vi "Motors help!.vi"(0 "Enable Motors":refnum<vi>, 1 "Cluster":T1, 2 "Motors Visa Ref":refnum<visa-resource-name>="COM7") -> ()   [LabVIEW 2010]
panel:
  out "theta-":refnum<vi>
  out "theta+":refnum<vi>
  out "Delta Theta (deg)":refnum<vi>
  out "Theta Speed (deg/s)":refnum<vi>
  out "theta-?":refnum<vi>
  out "theta+?":refnum<vi>
  out "Defined Positions":refnum<vi>
  out "Go To Saved Position?":refnum<vi>
  out "Saved Positions":refnum<vi>
  out "z-":refnum<vi>
  out "z+":refnum<vi>
  out "Delta Z (mm)":refnum<vi>
  out "Z Speed (mm/s)":refnum<vi>
  out "z-?":refnum<vi>
  out "z+?":refnum<vi>
  out "Y Speed (mm/s)":refnum<vi>
  out "y-":refnum<vi>
  out "y+":refnum<vi>
  out "Delta Y (mm)":refnum<vi>
  out "y-?":refnum<vi>
  out "y+?":refnum<vi>
  out "x-":refnum<vi>
  out "x+":refnum<vi>
  out "X Speed (mm/s)":refnum<vi>
  out "Delta X (mm)":refnum<vi>
  out "x-?":refnum<vi>
  out "x+?":refnum<vi>
  out "Jog-Mode":refnum<vi>
  out "Theta Go To":refnum<vi>
  out "Theta Go?":refnum<vi>
  out "Z Go To":refnum<vi>
  out "Z Go?":refnum<vi>
  out "Y Go To":refnum<vi>
  out "Y Go?":refnum<vi>
  out "X Go To":refnum<vi>
  out "X Go?":refnum<vi>
  out "Use Datums Nearest Hard Limits to Reset Origin?":refnum<vi>
  out "Saved Limits":refnum<vi>
  out "Find Datums Nearest Hard Limits?":refnum<vi>
  out "Theta Moving":refnum<vi>
  out "Status Theta":refnum<vi>
  out "Theta (deg)":refnum<vi>
  out "Theta Jogger Fast Speed":refnum<vi>
  out "Theta Jogger Normal Speed":refnum<vi>
  out "Theta Slew Speed (mm or degree/s)":refnum<vi>
  out "Z Moving":refnum<vi>
  out "Status Z":refnum<vi>
  out "Z-Axis (mm)":refnum<vi>
  out "Z Jogger Fast Speed":refnum<vi>
  out "Z Jogger Normal Speed":refnum<vi>
  out "Z Slew Speed (mm or degree/s)":refnum<vi>
  out "Y Moving":refnum<vi>
  out "Status Y":refnum<vi>
  out "Y-Axis (mm)":refnum<vi>
  out "Y Jogger Fast Speed":refnum<vi>
  out "Y Jogger Normal Speed":refnum<vi>
  out "Y Slew Speed (mm or degree/s)":refnum<vi>
  out "X Moving":refnum<vi>
  out "Status X":refnum<vi>
  out "X-Axis (mm)":refnum<vi>
  out "X Slew Speed (mm or degree/s)":refnum<vi>
  out "X Jogger Fast Speed":refnum<vi>
  out "X Jogger Normal Speed":refnum<vi>
  out "Set Jogger?":refnum<vi>
  out "Normal":refnum<vi>
  out "Fast":refnum<vi>
  out "Jogger Axis":refnum<vi>
  out "Theta Multiplier":refnum<vi>
  out "Z Multiplier":refnum<vi>
  out "Y Multiplier":refnum<vi>
  out "X Multiplier":refnum<vi>
  out "Need to Update Motor Parameters":refnum<vi>
  out "(degrees/s)":refnum<vi>
  out "Theta Set Slew Speed?":refnum<vi>
  out "(mm/s) 3":refnum<vi>
  out "Z Set Slew Speed?":refnum<vi>
  out "(mm/s) 2":refnum<vi>
  out "Y Set Slew Speed?":refnum<vi>
  out "(mm/s)":refnum<vi>
  out "X Set Slew Speed?":refnum<vi>
  out "Save Current Motor Parameters?":refnum<vi>
  out "Redefine Origin as Current Location?":refnum<vi>
  out "Reset Motors?":refnum<vi>
  out "Manual Communication is Active\n(Close Before Ending Program)":refnum<vi>
  out "Manual IO?":refnum<vi>
  out "EMERGENCY":refnum<vi>
  out "Backlash Theta":refnum<vi>
  out "Backlash Z":refnum<vi>
  out "Backlash Y":refnum<vi>
  out "Backlash X":refnum<vi>
  out "Backlash?":refnum<vi>
  out "Stop Theta?":refnum<vi>
  out "Stop Z?":refnum<vi>
  out "Stop Y?":refnum<vi>
  out "Stop X?":refnum<vi>
  in  "Enable Motors":bool
  out "Theta Action":string
  out "Z Action":string
  out "Y Action":string
  out "X Action":string
  in  "Steps to deactivate hard limit after finding datums":dbl=1000.0
  out "Loop i":i32
types:
  T1 = cluster{"Stop X?":refnum<vi>, "Stop Y?":refnum<vi>, "Stop Z?":refnum<vi>, "Stop Theta?":refnum<vi>, "Backlash?":refnum<vi>, "Backlash X":refnum<vi>, "Backlash Y":refnum<vi>, "Backlash Z":refnum<vi>, "Backlash Theta":refnum<vi>, "Manual IO?":refnum<vi>, "Manual Communication is Active\n(Close Before Ending Program)":refnum<vi>, "Reset Motors?":refnum<vi>, "Set Jogger?":refnum<vi>, "Normal":refnum<vi>, "Fast":refnum<vi>, "Jogger Axis":refnum<vi>, "Redefine Origin as Current Location?":refnum<vi>, "Save Current Motor Parameters?":refnum<vi>, "Find Datums Nearest Hard Limits?":refnum<vi>, "Saved Limits":refnum<vi>, "Use Datums Nearest Hard Limits to Reset Origin?":refnum<vi>, "X Go?":refnum<vi>, "Y Go?":refnum<vi>, "Z Go?":refnum<vi>, "Theta Go?":refnum<vi>, "Jog-Mode":refnum<vi>, "x+?":refnum<vi>, "x-?":refnum<vi>, "y+?":refnum<vi>, "y-?":refnum<vi>, "z+?":refnum<vi>, "z-?":refnum<vi>, "theta+?":refnum<vi>, "theta-?":refnum<vi>, "X Set Slew Speed?":refnum<vi>, "(mm/s)":refnum<vi>, "Y Set Slew Speed?":refnum<vi>, "(mm/s)":refnum<vi>, "Z Set Slew Speed?":refnum<vi>, "(mm/s)":refnum<vi>, "Theta Set Slew Speed?":refnum<vi>, "(degrees/s)":refnum<vi>, "Go To Saved Position?":refnum<vi>, "Defined Positions":refnum<vi>, "Need to Update Motor Parameters":refnum<vi>, "X Jogger Normal Speed":refnum<vi>, "X Jogger Fast Speed":refnum<vi>, "Y Jogger Normal Speed":refnum<vi>, "Y Jogger Fast Speed":refnum<vi>, "Z Jogger Normal Speed":refnum<vi>, "Z Jogger Fast Speed":refnum<vi>, "Theta Jogger Normal Speed":refnum<vi>, "Theta Jogger Fast Speed":refnum<vi>, "X Moving":refnum<vi>, "Y Moving":refnum<vi>, "Z Moving":refnum<vi>, "Theta Moving":refnum<vi>, "X Slew Speed (mm or degree/s)":refnum<vi>, "Y Slew Speed (mm or degree/s)":refnum<vi>, "Z Slew Speed (mm or degree/s)":refnum<vi>, "Theta Slew Speed (mm or degree/s)":refnum<vi>, "X-Axis (mm)":refnum<vi>, "Y-Axis (mm)":refnum<vi>, "Z-Axis (mm)":refnum<vi>, "Theta (deg)":refnum<vi>, "X Multiplier":refnum<vi>, "Y Multiplier":refnum<vi>, "Z Multiplier":refnum<vi>, "Theta Multiplier":refnum<vi>, "Motors Online":refnum<vi>, "Motors Status":refnum<vi>, "Status X":refnum<vi>, "Status Y":refnum<vi>, "Status Z":refnum<vi>, "Status Theta":refnum<vi>, "Motors error":refnum<vi>, "QUIT":refnum<vi>, "EMERGENCY":refnum<vi>, "X Go To":refnum<vi>, "Y Go To":refnum<vi>, "Z Go To":refnum<vi>, "Theta Go To":refnum<vi>, "Delta X (mm)":refnum<vi>, "Delta Y (mm)":refnum<vi>, "Delta Z (mm)":refnum<vi>, "Delta Theta (deg)":refnum<vi>, "X Speed (mm/s)":refnum<vi>, "Y Speed (mm/s)":refnum<vi>, "Z Speed (mm/s)":refnum<vi>, "Theta Speed (deg/s)":refnum<vi>, "x+":refnum<vi>, "x-":refnum<vi>, "y+":refnum<vi>, "y-":refnum<vi>, "z+":refnum<vi>, "z-":refnum<vi>, "theta+":refnum<vi>, "theta-":refnum<vi>, "Saved Positions":refnum<vi>}
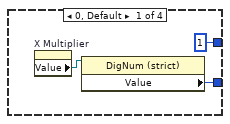
[diagram p3: hidden frame]
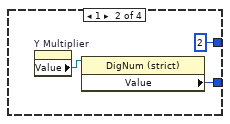
[diagram p4: hidden frame]
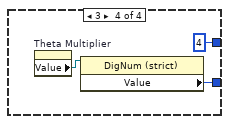
[diagram p5: hidden frame]
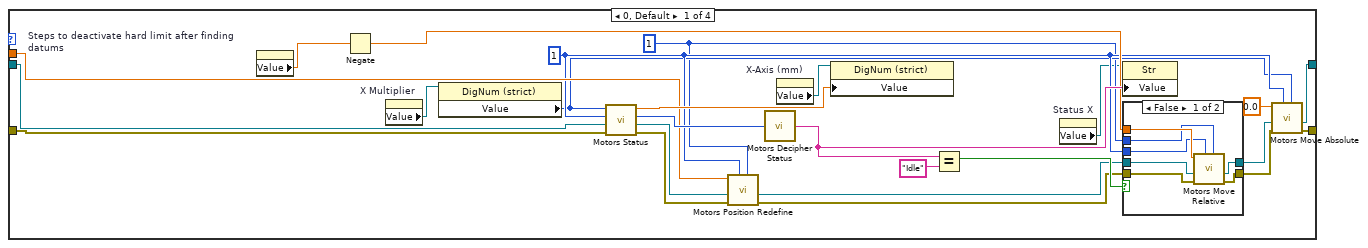
[diagram p15: hidden frame]
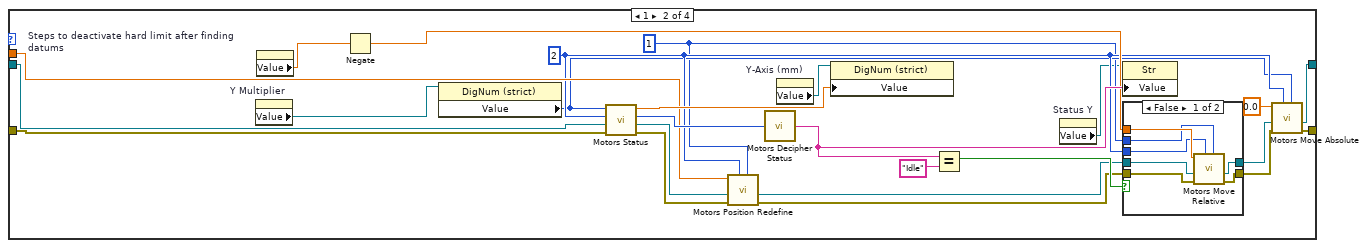
[diagram p17: hidden frame]
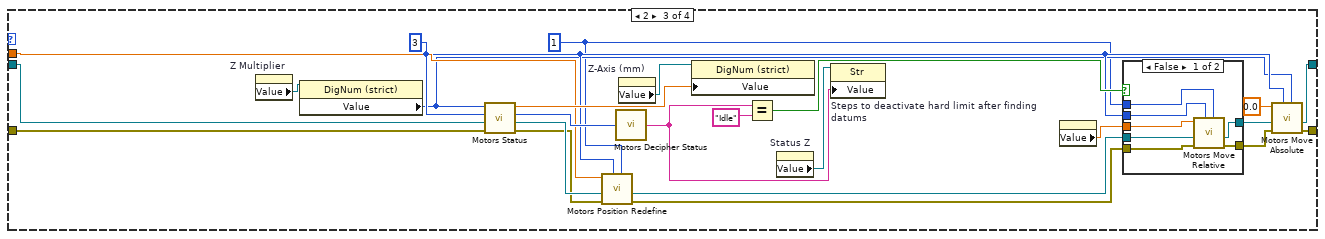
[diagram p19: hidden frame]
diagram:
  n1 = call "Motors Open.vi"("VISA in"="Motors Visa Ref") -> ("error out"=w111:errorcluster, "VISA out"=w2:refnum<visa-resource-name>)  [unwired: 1 in]
  n2 = call <vilib>:"Simple Error Handler.vi"("error in (no error)"=w111) -> ("error?"=w110:bool, "error out"=w112:errorcluster)  [unwired: 4 in, 3 out]
  n3 = Unbundle("Cluster") -> ("Stop X?"=→"Stop X?":refnum<vi>, "Stop Y?"=→"Stop Y?":refnum<vi>, "Stop Z?"=→"Stop Z?":refnum<vi>, "Stop Theta?"=→"Stop Theta?":refnum<vi>, "Backlash?"=→"Backlash?":refnum<vi>, "Backlash X"=→"Backlash X":refnum<vi>, "Backlash Y"=→"Backlash Y":refnum<vi>, "Backlash Z"=→"Backlash Z":refnum<vi>, "Backlash Theta"=→"Backlash Theta":refnum<vi>, "Manual IO?"=→"Manual IO?":refnum<vi>, "Manual Communication is Active\n(Close Before Ending Program)"=→"Manual Communication is Active\n(Close Before Ending Program)":refnum<vi>, "Reset Motors?"=→"Reset Motors?":refnum<vi>, "Set Jogger?"=→"Set Jogger?":refnum<vi>, "Normal"=→"Normal":refnum<vi>, "Fast"=→"Fast":refnum<vi>, "Jogger Axis"=→"Jogger Axis":refnum<vi>, "Redefine Origin as Current Location?"=→"Redefine Origin as Current Location?":refnum<vi>, "Save Current Motor Parameters?"=→"Save Current Motor Parameters?":refnum<vi>, "Find Datums Nearest Hard Limits?"=→"Find Datums Nearest Hard Limits?":refnum<vi>, "Saved Limits"=→"Saved Limits":refnum<vi>, "Use Datums Nearest Hard Limits to Reset Origin?"=→"Use Datums Nearest Hard Limits to Reset Origin?":refnum<vi>, "X Go?"=→"X Go?":refnum<vi>, "Y Go?"=→"Y Go?":refnum<vi>, "Z Go?"=→"Z Go?":refnum<vi>, "Theta Go?"=→"Theta Go?":refnum<vi>, "Jog-Mode"=→"Jog-Mode":refnum<vi>, "x+?"=→"x+?":refnum<vi>, "x-?"=→"x-?":refnum<vi>, "y+?"=→"y+?":refnum<vi>, "y-?"=→"y-?":refnum<vi>, "z+?"=→"z+?":refnum<vi>, "z-?"=→"z-?":refnum<vi>, "theta+?"=→"theta+?":refnum<vi>, "theta-?"=→"theta-?":refnum<vi>, "X Set Slew Speed?"=→"X Set Slew Speed?":refnum<vi>, "(mm/s)"=→"(mm/s)":refnum<vi>, "Y Set Slew Speed?"=→"Y Set Slew Speed?":refnum<vi>, "(mm/s)"=→"(mm/s) 2":refnum<vi>, "Z Set Slew Speed?"=→"Z Set Slew Speed?":refnum<vi>, "(mm/s)"=→"(mm/s) 3":refnum<vi>, "Theta Set Slew Speed?"=→"Theta Set Slew Speed?":refnum<vi>, "(degrees/s)"=→"(degrees/s)":refnum<vi>, "Go To Saved Position?"=→"Go To Saved Position?":refnum<vi>, "Defined Positions"=→"Defined Positions":refnum<vi>, "Need to Update Motor Parameters"=w5:refnum<vi>, "X Jogger Normal Speed"=→"X Jogger Normal Speed":refnum<vi>, "X Jogger Fast Speed"=→"X Jogger Fast Speed":refnum<vi>, "Y Jogger Normal Speed"=→"Y Jogger Normal Speed":refnum<vi>, "Y Jogger Fast Speed"=→"Y Jogger Fast Speed":refnum<vi>, "Z Jogger Normal Speed"=→"Z Jogger Normal Speed":refnum<vi>, "Z Jogger Fast Speed"=→"Z Jogger Fast Speed":refnum<vi>, "Theta Jogger Normal Speed"=→"Theta Jogger Normal Speed":refnum<vi>, "Theta Jogger Fast Speed"=→"Theta Jogger Fast Speed":refnum<vi>, "X Moving"=→"X Moving":refnum<vi>, "Y Moving"=→"Y Moving":refnum<vi>, "Z Moving"=→"Z Moving":refnum<vi>, "Theta Moving"=→"Theta Moving":refnum<vi>, "X Slew Speed (mm or degree/s)"=→"X Slew Speed (mm or degree/s)":refnum<vi>, "Y Slew Speed (mm or degree/s)"=→"Y Slew Speed (mm or degree/s)":refnum<vi>, "Z Slew Speed (mm or degree/s)"=→"Z Slew Speed (mm or degree/s)":refnum<vi>, "Theta Slew Speed (mm or degree/s)"=→"Theta Slew Speed (mm or degree/s)":refnum<vi>, "X-Axis (mm)"=→"X-Axis (mm)":refnum<vi>, "Y-Axis (mm)"=→"Y-Axis (mm)":refnum<vi>, "Z-Axis (mm)"=→"Z-Axis (mm)":refnum<vi>, "Theta (deg)"=→"Theta (deg)":refnum<vi>, "X Multiplier"=→"X Multiplier":refnum<vi>, "Y Multiplier"=→"Y Multiplier":refnum<vi>, "Z Multiplier"=→"Z Multiplier":refnum<vi>, "Theta Multiplier"=→"Theta Multiplier":refnum<vi>, "Motors Online"=w88:refnum<vi>, "Motors Status"=w89:refnum<vi>, "Status X"=→"Status X":refnum<vi>, "Status Y"=→"Status Y":refnum<vi>, "Status Z"=→"Status Z":refnum<vi>, "Status Theta"=→"Status Theta":refnum<vi>, "Motors error"=w16:refnum<vi>, "QUIT"=w108:refnum<vi>, "EMERGENCY"=→"EMERGENCY":refnum<vi>, "X Go To"=→"X Go To":refnum<vi>, "Y Go To"=→"Y Go To":refnum<vi>, "Z Go To"=→"Z Go To":refnum<vi>, "Theta Go To"=→"Theta Go To":refnum<vi>, "Delta X (mm)"=→"Delta X (mm)":refnum<vi>, "Delta Y (mm)"=→"Delta Y (mm)":refnum<vi>, "Delta Z (mm)"=→"Delta Z (mm)":refnum<vi>, "Delta Theta (deg)"=→"Delta Theta (deg)":refnum<vi>, "X Speed (mm/s)"=→"X Speed (mm/s)":refnum<vi>, "Y Speed (mm/s)"=→"Y Speed (mm/s)":refnum<vi>, "Z Speed (mm/s)"=→"Z Speed (mm/s)":refnum<vi>, "Theta Speed (deg/s)"=→"Theta Speed (deg/s)":refnum<vi>, "x+"=→"x+":refnum<vi>, "x-"=→"x-":refnum<vi>, "y+"=→"y+":refnum<vi>, "y-"=→"y-":refnum<vi>, "z+"=→"z+":refnum<vi>, "z-"=→"z-":refnum<vi>, "theta+"=→"theta+":refnum<vi>, "theta-"=→"theta-":refnum<vi>, "Saved Positions"=→"Saved Positions":refnum<vi>)
  "Need to Update Motor Parameters" <- w5
  n4 = property on="Property Node" class="Clust (strict)"(reference=w16, "Value"=w112) -> ()  [unwired: 1 in, 2 out]
  n5 = property on="Property Node" class="Bool (strict)"(reference=w5, "Value"=TRUE) -> ()  [unwired: 1 in, 2 out]
  n6 = Not(x=w110) -> (.not. x?=w109:bool)
  n7 = property on="Property Node" class="Bool (strict)"(reference=w88, "Value"=w109) -> ()  [unwired: 1 in, 2 out]
  n8 = property on="Property Node" class="Str"(reference=w89, "Value"="Opening Communication Channels") -> (reference out=w107:refnum<vi>)  [unwired: 1 in, 1 out]
  n9 = case shown="True" w109 {
    tunnel: w107 -> [_ w120]
    tunnel: w2 -> [w114 w119]
    tunnel: w16 -> [_ w118]
    tunnel: w108 -> [_ w117]
    tunnel: [w114 w115] -> w1
    frame False {
    }
    frame True {
      n10 = property on="Property Node" class="Str"(reference=w120, "Value"="Running") -> (reference out=w116:refnum<vi>)  [unwired: 1 in, 1 out]
      n11 = while {
        shift-right: [w122] -> w115
        shift-left: w119 -> [w208]
        tunnel: w118 -> [w166]
        tunnel: w117 -> [w245]
        tunnel: w116 -> [w242]
        i -> [w246]
        stop <- w164 stop-if-true
        # "This loop contains all of the code that has to communicate directly with the manipulator motor controllers.  They are arranged linearly to ensure multiple serial I/O's are never attempted simultaneously.  Note that this loop executes very slowly (each serial I/O takes about 1/20 sec).\n\nWarning: Pushing LabView's \"Clean Up Diagram\" button will likely cause LabView to crash (because this VI is way too big)."
        n12 = property on="Stop X?" class="LVObjRef (strict)"() -> ("Value"=w160:refnum<vi>)  [unwired: 2 in, 2 out]
        n13 = property on="Reset Motors?" class="LVObjRef (strict)"() -> ("Value"=w154:refnum<vi>)  [unwired: 2 in, 2 out]
        n14 = property on="Property Node" class="Bool (strict)"(reference="Enable Motors") -> ("Value"=w162:bool)  [unwired: 1 in, 2 out]
        n15 = property on="Property Node" class="Bool (strict)"(reference=w160) -> (reference out=w222:refnum<vi>, "Value"=w215:bool)  [unwired: 1 in, 1 out]
        n16 = property on="Property Node" class="Bool (strict)"(reference=w154) -> (reference out=w202:refnum<vi>, "Value"=w201:bool)  [unwired: 1 in, 1 out]
        n17 = property on="Property Node" class="Clust (strict)"(reference=w166) -> (reference out=w124:refnum<vi>, "Value"=w207:errorcluster)  [unwired: 1 in, 1 out]
        n18 = Not(x=w162) -> (.not. x?=w161:bool)
        n19 = property on="Property Node" class="Bool (strict)"(reference=w245) -> ("Value"=w165:bool)  [unwired: 1 in, 2 out]
        n20 = case shown="True" w215 {
          tunnel: w207 -> [w400 w408]
          tunnel: w208 -> [w401 w407]
          tunnel: [w401 w405] -> w214
          tunnel: [w400 w404] -> w213
          tunnel: w222 -> [_ w402]
          frame False {
          }
          frame True {
            n21 = property on="Property Node" class="Bool (strict)"(reference=w402, "Value"=FALSE) -> ()  [unwired: 1 in, 2 out]
            n22 = call "Motors Stop.vi"("error in"=w408, "Axis"=1, "VISA in"=w407) -> ("error out"=w404:errorcluster, "VISA out"=w405:refnum<visa-resource-name>)
          }
        }
        n23 = Or(x=w165, y=w161) -> (x .or. y?=w164:bool)
        n24 = property on="Stop Y?" class="LVObjRef (strict)"() -> ("Value"=w159:refnum<vi>)  [unwired: 2 in, 2 out]
        n25 = property on="Property Node" class="Bool (strict)"(reference=w159) -> (reference out=w221:refnum<vi>, "Value"=w216:bool)  [unwired: 1 in, 1 out]
        n26 = case shown="True" w216 {
          tunnel: w213 -> [w391 w399]
          tunnel: w214 -> [w392 w398]
          tunnel: [w392 w396] -> w212
          tunnel: [w391 w395] -> w211
          tunnel: w221 -> [_ w393]
          frame False {
          }
          frame True {
            n27 = property on="Property Node" class="Bool (strict)"(reference=w393, "Value"=FALSE) -> ()  [unwired: 1 in, 2 out]
            n28 = call "Motors Stop.vi"("error in"=w399, "Axis"=2, "VISA in"=w398) -> ("error out"=w395:errorcluster, "VISA out"=w396:refnum<visa-resource-name>)
          }
        }
        n29 = property on="Stop Z?" class="LVObjRef (strict)"() -> ("Value"=w158:refnum<vi>)  [unwired: 2 in, 2 out]
        n30 = property on="Property Node" class="Bool (strict)"(reference=w158) -> (reference out=w220:refnum<vi>, "Value"=w217:bool)  [unwired: 1 in, 1 out]
        n31 = case shown="True" w217 {
          tunnel: w211 -> [w382 w390]
          tunnel: w212 -> [w383 w389]
          tunnel: [w383 w387] -> w210
          tunnel: [w382 w386] -> w209
          tunnel: w220 -> [_ w384]
          frame False {
          }
          frame True {
            n32 = property on="Property Node" class="Bool (strict)"(reference=w384, "Value"=FALSE) -> ()  [unwired: 1 in, 2 out]
            n33 = call "Motors Stop.vi"("error in"=w390, "Axis"=3, "VISA in"=w389) -> ("error out"=w386:errorcluster, "VISA out"=w387:refnum<visa-resource-name>)
          }
        }
        n34 = property on="Stop Theta?" class="LVObjRef (strict)"() -> ("Value"=w157:refnum<vi>)  [unwired: 2 in, 2 out]
        n35 = property on="Property Node" class="Bool (strict)"(reference=w157) -> (reference out=w219:refnum<vi>, "Value"=w218:bool)  [unwired: 1 in, 1 out]
        n36 = case shown="True" w218 {
          tunnel: w209 -> [w373 w381]
          tunnel: w210 -> [w374 w380]
          tunnel: [w374 w378] -> w203
          tunnel: [w373 w377] -> w204
          tunnel: w219 -> [_ w375]
          frame False {
          }
          frame True {
            n37 = property on="Property Node" class="Bool (strict)"(reference=w375, "Value"=FALSE) -> ()  [unwired: 1 in, 2 out]
            n38 = call "Motors Stop.vi"("error in"=w381, "Axis"=4, "VISA in"=w380) -> ("error out"=w377:errorcluster, "VISA out"=w378:refnum<visa-resource-name>)
          }
        }
        n39 = property on="Backlash?" class="LVObjRef (strict)"() -> ("Value"=w156:refnum<vi>)  [unwired: 2 in, 2 out]
        n40 = property on="Property Node" class="Bool (strict)"(reference=w156) -> (reference out=w206:refnum<vi>, "Value"=w205:bool)  [unwired: 1 in, 1 out]
        n41 = case shown="True" w205 {
          tunnel: [w358 w372] -> w196
          tunnel: w206 -> [_ w366]
          tunnel: w203 -> [w358 w365]
          tunnel: w204 -> [w357 w364]
          tunnel: [w357 w363] -> w195
          frame False {
          }
          frame True {
            n42 = property on="Property Node" class="Bool (strict)"(reference=w366, "Value"=FALSE) -> ()  [unwired: 1 in, 2 out]
            n43 = property on="Backlash X" class="LVObjRef (strict)"() -> ("Value"=w362:refnum<vi>)  [unwired: 2 in, 2 out]
            n44 = property on="Backlash Z" class="LVObjRef (strict)"() -> ("Value"=w360:refnum<vi>)  [unwired: 2 in, 2 out]
            n45 = property on="Backlash Y" class="LVObjRef (strict)"() -> ("Value"=w361:refnum<vi>)  [unwired: 2 in, 2 out]
            n46 = property on="Backlash Theta" class="LVObjRef (strict)"() -> ("Value"=w359:refnum<vi>)  [unwired: 2 in, 2 out]
            n47 = property on="Property Node" class="DigNum (strict)"(reference=w362) -> ("Value"=w371:u32)  [unwired: 1 in, 2 out]
            n48 = property on="Property Node" class="DigNum (strict)"(reference=w359) -> ("Value"=w368:u32)  [unwired: 1 in, 2 out]
            n49 = property on="Property Node" class="DigNum (strict)"(reference=w360) -> ("Value"=w369:u32)  [unwired: 1 in, 2 out]
            n50 = property on="Property Node" class="DigNum (strict)"(reference=w361) -> ("Value"=w370:u32)  [unwired: 1 in, 2 out]
            n51 = call "Motors Backlash.vi"("X"=w371, "Y"=w370, "VISA in"=w365, "error in"=w364, "Z"=w369, "Theta"=w368) -> ("VISA out"=w372:refnum<visa-resource-name>, "error out"=w363:errorcluster)  [unwired: 2 in]
          }
        }
        n52 = property on="Manual IO?" class="LVObjRef (strict)"() -> ("Value"=w155:refnum<vi>)  [unwired: 2 in, 2 out]
        n53 = property on="Property Node" class="Bool (strict)"(reference=w155) -> (reference out=w200:refnum<vi>, "Value"=w199:bool)  [unwired: 1 in, 1 out]
        n54 = case shown="True" w199 {
          tunnel: [w332 w343] -> w198
          tunnel: [w333 w335] -> w197
          tunnel: w200 -> [_ w337]
          tunnel: w196 -> [w333 w336]
          tunnel: w195 -> [w332 w334]
          frame False {
          }
          frame True {
            n55 = flat-sequence {
              tunnel: [w345] -> w339
              tunnel: [w352] -> w342
              tunnel: [w351] -> w341
              tunnel: [w350] -> w340
              tunnel: w339 -> [w350]
              tunnel: w336 -> [w349]
              tunnel: w334 -> [w348]
              tunnel: [w355] -> w335
              tunnel: [w356] -> w343
              tunnel: w342 -> [w356]
              tunnel: w341 -> [w355]
              tunnel: w340 -> [w353]
              frame #0 {
                n56 = property on="Manual Communication is Active\n(Close Before Ending Program)" class="LVObjRef (strict)"() -> ("Value"=w344:refnum<vi>)  [unwired: 2 in, 2 out]
                n57 = property on="Property Node" class="Bool (strict)"(reference=w344, "Value"=TRUE ("Manual Communication is Active\n(Close Before Ending Program) 2")) -> (reference out=w345:refnum<vi>)  [unwired: 1 in, 1 out]
              }
              frame #1 {
                n58 = property on="EMERGENCY" class="LVObjRef (strict)"() -> ("Value"=w347:refnum<vi>)  [unwired: 2 in, 2 out]
                n59 = call "Motors Manual IO.vi"("error in"=w348, "Emergency Stop Reference"=w347, "VISA in"=w349) -> ("error out"=w352:errorcluster, "VISA out"=w351:refnum<visa-resource-name>)
              }
              frame #2 {
                n60 = property on="Property Node" class="Bool (strict)"(reference=w353, "Value"=FALSE ("Manual Communication is Active\n(Close Before Ending Program)")) -> ()  [unwired: 1 in, 2 out]
              }
            }
            n61 = property on="Property Node" class="Bool (strict)"(reference=w337, "Value"=FALSE) -> ()  [unwired: 1 in, 2 out]
          }
        }
        n62 = property on="Jogger Axis" class="LVObjRef (strict)"() -> ("Value"=w146:refnum<vi>)  [unwired: 2 in, 2 out]
        n63 = property on="Property Node" class="Ring (strict)"(reference=w146) -> ("Value"=w194:u16)  [unwired: 1 in, 2 out]
        n64 = case shown="2" w194 {
          tunnel: [u32 1 u32 2 u32 3 u32 4] -> _
          tunnel: [w298 w301 w304 w307] -> w193
          frame 0, Default {
            n65 = property on="X Multiplier" class="LVObjRef (strict)"() -> ("Value"=w297:refnum<vi>)  [unwired: 2 in, 2 out]
            n66 = property on="Property Node" class="DigNum (strict)"(reference=w297) -> ("Value"=w298:u32)  [unwired: 1 in, 2 out]
          }
          frame 1 {
            n67 = property on="Y Multiplier" class="LVObjRef (strict)"() -> ("Value"=w300:refnum<vi>)  [unwired: 2 in, 2 out]
            n68 = property on="Property Node" class="DigNum (strict)"(reference=w300) -> ("Value"=w301:u32)  [unwired: 1 in, 2 out]
          }
          frame 2 {
            n69 = property on="Z Multiplier" class="LVObjRef (strict)"() -> ("Value"=w303:refnum<vi>)  [unwired: 2 in, 2 out]
            n70 = property on="Property Node" class="DigNum (strict)"(reference=w303) -> ("Value"=w304:u32)  [unwired: 1 in, 2 out]
          }
          frame 3 {
            n71 = property on="Theta Multiplier" class="LVObjRef (strict)"() -> ("Value"=w306:refnum<vi>)  [unwired: 2 in, 2 out]
            n72 = property on="Property Node" class="DigNum (strict)"(reference=w306) -> ("Value"=w307:u32)  [unwired: 1 in, 2 out]
          }
        }
        n73 = case shown="True" w201 {
          tunnel: [w324 w331] -> w189
          tunnel: [w325 w330] -> w190
          tunnel: w197 -> [w325 w329]
          tunnel: w198 -> [w324 w328]
          tunnel: w202 -> [_ w326]
          frame False {
          }
          frame True {
            n74 = property on="Property Node" class="Bool (strict)"(reference=w326, "Value"=FALSE) -> ()  [unwired: 1 in, 2 out]
            n75 = call "Motors Reset.vi"("error in"=w328, "VISA in"=w329) -> ("error out"=w331:errorcluster, "VISA out"=w330:refnum<visa-resource-name>)
          }
        }
        n76 = property on="Set Jogger?" class="LVObjRef (strict)"() -> ("Value"=w147:refnum<vi>)  [unwired: 2 in, 2 out]
        n77 = property on="Property Node" class="Bool (strict)"(reference=w147) -> (reference out=w192:refnum<vi>, "Value"=w191:bool)  [unwired: 1 in, 1 out]
        n78 = case shown="True" w191 {
          tunnel: [w310 w323] -> w187
          tunnel: [w309 w321] -> w188
          tunnel: w193 -> [_ w322]
          tunnel: w192 -> [_ w319]
          tunnel: w189 -> [w310 w315]
          tunnel: w190 -> [w309 w314]
          frame False {
          }
          frame True {
            n79 = property on="Property Node" class="Bool (strict)"(reference=w319, "Value"=FALSE ("Need to Update Motor Parameters")) -> ()  [unwired: 1 in, 2 out]
            n80 = property on="Normal" class="LVObjRef (strict)"() -> ("Value"=w312:refnum<vi>)  [unwired: 2 in, 2 out]
            n81 = property on="Need to Update Motor Parameters" class="LVObjRef (strict)"() -> ("Value"=w311:refnum<vi>)  [unwired: 2 in, 2 out]
            n82 = property on="Fast" class="LVObjRef (strict)"() -> ("Value"=w313:refnum<vi>)  [unwired: 2 in, 2 out]
            n83 = property on="Property Node" class="DigNum (strict)"(reference=w312) -> ("Value"=w318:dbl)  [unwired: 1 in, 2 out]
            n84 = property on="Property Node" class="DigNum (strict)"(reference=w313) -> ("Value"=w317:dbl)  [unwired: 1 in, 2 out]
            n85 = property on="Property Node" class="Bool (strict)"(reference=w311, "Value"=TRUE) -> ()  [unwired: 1 in, 2 out]
            n86 = call "Motors Jogger Speed.vi"("Axis Multiplier"=w322, "error in"=w315, "VISA in"=w314, "Fast Speed (mm or degree/sec)"=w317, "Normal Speed (mm or degree/sec)"=w318) -> ("error out"=w323:errorcluster, "VISA out"=w321:refnum<visa-resource-name>)  [unwired: 5 in]
          }
        }
        n87 = property on="Redefine Origin as Current Location?" class="LVObjRef (strict)"() -> ("Value"=w153:refnum<vi>)  [unwired: 2 in, 2 out]
        n88 = property on="Property Node" class="Bool (strict)"(reference=w153) -> (reference out=w234:refnum<vi>, "Value"=w244:bool)  [unwired: 1 in, 1 out]
        n89 = case shown="True" w244 {
          tunnel: w188 -> [w1407 w1414]
          tunnel: w187 -> [w1408 w1410]
          tunnel: [w1408 w1412] -> w237
          tunnel: [w1407 w1413] -> w296
          tunnel: w234 -> [_ w1409]
          frame False {
          }
          frame True {
            n90 = property on="Property Node" class="Bool (strict)"(reference=w1409, "Value"=FALSE) -> ()  [unwired: 1 in, 2 out]
            n91 = call "Motors Redefine Origin.vi"("error in"=w1410, "VISA in"=w1414) -> ("error out"=w1412:errorcluster, "VISA out"=w1413:refnum<visa-resource-name>)
          }
        }
        n92 = property on="Save Current Motor Parameters?" class="LVObjRef (strict)"() -> ("Value"=w152:refnum<vi>)  [unwired: 2 in, 2 out]
        n93 = property on="Property Node" class="Bool (strict)"(reference=w152) -> (reference out=w236:refnum<vi>, "Value"=w235:bool)  [unwired: 1 in, 1 out]
        n94 = case shown="True" w235 {
          tunnel: w237 -> [w1400 w1406]
          tunnel: [w1400 w1405] -> w252
          tunnel: w296 -> [w1399 w1404]
          tunnel: [w1399 w1403] -> w251
          tunnel: w236 -> [_ w1402]
          frame False {
          }
          frame True {
            n95 = property on="Property Node" class="Bool (strict)"(reference=w1402, "Value"=FALSE) -> ()  [unwired: 1 in, 2 out]
            n96 = call "Motors Save.vi"("error in"=w1406, "VISA in"=w1404) -> ("error out"=w1405:errorcluster, "VISA out"=w1403:refnum<visa-resource-name>)
          }
        }
        n97 = property on="Find Datums Nearest Hard Limits?" class="LVObjRef (strict)"() -> ("Value"=w144:refnum<vi>)  [unwired: 2 in, 2 out]
        n98 = property on="Property Node" class="Bool (strict)"(reference=w144) -> (reference out=w238:refnum<vi>, "Value"=w243:bool)  [unwired: 1 in, 1 out]
        n99 = case shown="True" w243 {
          tunnel: w252 -> [w588 w601]
          tunnel: [w588 w599] -> w249
          tunnel: [w587 w600] -> w247
          tunnel: w251 -> [w587 w602]
          tunnel: w242 -> [w586 w594]
          tunnel: [w586 w591] -> w240
          tunnel: w238 -> [_ w590]
          frame False {
          }
          frame True {
            n100 = property on="Property Node" class="Bool (strict)"(reference=w590, "Value"=FALSE) -> ()  [unwired: 1 in, 2 out]
            n101 = flat-sequence {
              tunnel: w601 -> [w607]
              tunnel: w602 -> [w608]
              tunnel: [w608] -> w598
              tunnel: [w607] -> w597
              tunnel: w594 -> [w604]
              tunnel: [w603] -> w592
              tunnel: w598 -> [w627]
              tunnel: w597 -> [w626]
              tunnel: [w622] -> w596
              tunnel: [w621] -> w595
              tunnel: [w611] -> w593
              tunnel: w592 -> [w611]
              tunnel: [w721] -> w599
              tunnel: [w722] -> w600
              tunnel: w596 -> [w722]
              tunnel: w595 -> [w721]
              tunnel: w593 -> [w719]
              tunnel: [w718] -> w591
              frame #0 {
                n102 = call <vilib>:"Set Busy.vi"("disable click? (T)"=FALSE) -> ()  [unwired: 9 in, 2 out]
                n103 = property on="Property Node" class="Str"(reference=w604, "Value"="Finding Datums Nearest Hard Limits\nThis May Take a Few Minutes" ("Status")) -> (reference out=w603:refnum<vi>)  [unwired: 1 in, 1 out]
              }
              frame #1 {
                n104 = call "Motors Find Datums.vi"("error in"=w626, "VISA in"=w627) -> ("error out"=w623:errorcluster, "VISA out"=w624:refnum<visa-resource-name>)
                n105 = for {
                  N: 4 -> [_]
                  shift-right: [w631] -> w621
                  shift-left: w623 -> [w632]
                  shift-right: [w630] -> w622
                  shift-left: w624 -> [w633]
                  tunnel: [w629] -> w613 mode=indexing
                  i -> [w628]
                  n106 = case shown="3" w628 {
                    tunnel: w632 -> [w646 w667 w688 w709]
                    tunnel: w633 -> [w647 w668 w689 w710]
                    tunnel: [w640 w661 w681 w702] -> w631
                    tunnel: [w641 w662 w682 w703] -> w630
                    tunnel: [w638 w659 w685 w706] -> w629
                    frame 0, Default {
                      w639 = 1 ("Axis")
                      n107 = property on="X Multiplier" class="LVObjRef (strict)"() -> ("Value"=w634:refnum<vi>)  [unwired: 2 in, 2 out]
                      n108 = property on="Property Node" class="DigNum (strict)"(reference=w634) -> ("Value"=w645:u32)  [unwired: 1 in, 2 out]
                      n109 = call "Motors Status.vi"("error in"=w646, "VISA in"=w647, "Axis"=w639, "Axis Multiplier"=w645) -> ("error out"=w642:errorcluster, "VISA out"=w643:refnum<visa-resource-name>, "OS"=w652:i32, "Actual Position (mm or deg)"=w644:dbl)  [unwired: 3 in]
                      n110 = call "Motors Datum Position.vi"("error in"=w642, "VISA in"=w643, "Axis"=w639) -> ("error out"=w640:errorcluster, "VISA out"=w641:refnum<visa-resource-name>, "Datum Position (steps)"=w638:string)  [unwired: 5 in]
                      n111 = call "Motors Decipher Status.vi"("OS"=w652) -> ("Status"=w651:string)
                      n112 = property on="X-Axis (mm)" class="LVObjRef (strict)"() -> ("Value"=w636:refnum<vi>)  [unwired: 2 in, 2 out]
                      n113 = property on="Property Node" class="DigNum (strict)"(reference=w636, "Value"=w644) -> ()  [unwired: 1 in, 2 out]
                      n114 = Equal?(x=w651, y="Idle") -> (x = y?=w649:bool)
                      n115 = property on="Status X" class="LVObjRef (strict)"() -> ("Value"=w637:refnum<vi>)  [unwired: 2 in, 2 out]
                      n116 = case shown="False" w649 {
                        tunnel: [TRUE FALSE] -> w648
                        frame False {
                        }
                        frame True {
                        }
                      }
                      n117 = property on="Property Node" class="Str"(reference=w637, "Value"=w651) -> ()  [unwired: 1 in, 2 out]
                      n118 = property on="X Moving" class="LVObjRef (strict)"() -> ("Value"=w635:refnum<vi>)  [unwired: 2 in, 2 out]
                      n119 = property on="Property Node" class="Bool (strict)"(reference=w635, "Value"=w648) -> ()  [unwired: 1 in, 2 out]
                    }
                    frame 1 {
                      w660 = 2 ("Axis")
                      n120 = property on="Y Multiplier" class="LVObjRef (strict)"() -> ("Value"=w658:refnum<vi>)  [unwired: 2 in, 2 out]
                      n121 = property on="Property Node" class="DigNum (strict)"(reference=w658) -> ("Value"=w666:u32)  [unwired: 1 in, 2 out]
                      n122 = call "Motors Status.vi"("error in"=w667, "VISA in"=w668, "Axis"=w660, "Axis Multiplier"=w666) -> ("error out"=w663:errorcluster, "VISA out"=w664:refnum<visa-resource-name>, "OS"=w673:i32, "Actual Position (mm or deg)"=w665:dbl)  [unwired: 3 in]
                      n123 = call "Motors Datum Position.vi"("error in"=w663, "VISA in"=w664, "Axis"=w660) -> ("error out"=w661:errorcluster, "VISA out"=w662:refnum<visa-resource-name>, "Datum Position (steps)"=w659:string)  [unwired: 5 in]
                      n124 = call "Motors Decipher Status.vi"("OS"=w673) -> ("Status"=w671:string)
                      n125 = property on="Y-Axis (mm)" class="LVObjRef (strict)"() -> ("Value"=w655:refnum<vi>)  [unwired: 2 in, 2 out]
                      n126 = property on="Property Node" class="DigNum (strict)"(reference=w655, "Value"=w665) -> ()  [unwired: 1 in, 2 out]
                      n127 = Equal?(x=w671, y="Idle") -> (x = y?=w670:bool)
                      n128 = property on="Status Y" class="LVObjRef (strict)"() -> ("Value"=w657:refnum<vi>)  [unwired: 2 in, 2 out]
                      n129 = case shown="False" w670 {
                        tunnel: [TRUE FALSE] -> w669
                        frame False {
                        }
                        frame True {
                        }
                      }
                      n130 = property on="Property Node" class="Str"(reference=w657, "Value"=w671) -> ()  [unwired: 1 in, 2 out]
                      n131 = property on="Y Moving" class="LVObjRef (strict)"() -> ("Value"=w656:refnum<vi>)  [unwired: 2 in, 2 out]
                      n132 = property on="Property Node" class="Bool (strict)"(reference=w656, "Value"=w669) -> ()  [unwired: 1 in, 2 out]
                    }
                    frame 2 {
                      w680 = 3 ("Axis")
                      n133 = property on="Z Multiplier" class="LVObjRef (strict)"() -> ("Value"=w679:refnum<vi>)  [unwired: 2 in, 2 out]
                      n134 = property on="Property Node" class="DigNum (strict)"(reference=w679) -> ("Value"=w687:u32)  [unwired: 1 in, 2 out]
                      n135 = call "Motors Status.vi"("error in"=w688, "VISA in"=w689, "Axis"=w680, "Axis Multiplier"=w687) -> ("error out"=w683:errorcluster, "VISA out"=w684:refnum<visa-resource-name>, "OS"=w694:i32, "Actual Position (mm or deg)"=w686:dbl)  [unwired: 3 in]
                      n136 = call "Motors Datum Position.vi"("error in"=w683, "VISA in"=w684, "Axis"=w680) -> ("error out"=w681:errorcluster, "VISA out"=w682:refnum<visa-resource-name>, "Datum Position (steps)"=w685:string)  [unwired: 5 in]
                      n137 = call "Motors Decipher Status.vi"("OS"=w694) -> ("Status"=w692:string)
                      n138 = property on="Z-Axis (mm)" class="LVObjRef (strict)"() -> ("Value"=w676:refnum<vi>)  [unwired: 2 in, 2 out]
                      n139 = property on="Property Node" class="DigNum (strict)"(reference=w676, "Value"=w686) -> ()  [unwired: 1 in, 2 out]
                      n140 = Equal?(x=w692, y="Idle") -> (x = y?=w691:bool)
                      n141 = property on="Status Z" class="LVObjRef (strict)"() -> ("Value"=w678:refnum<vi>)  [unwired: 2 in, 2 out]
                      n142 = case shown="False" w691 {
                        tunnel: [TRUE FALSE] -> w690
                        frame False {
                        }
                        frame True {
                        }
                      }
                      n143 = property on="Property Node" class="Str"(reference=w678, "Value"=w692) -> ()  [unwired: 1 in, 2 out]
                      n144 = property on="Z Moving" class="LVObjRef (strict)"() -> ("Value"=w677:refnum<vi>)  [unwired: 2 in, 2 out]
                      n145 = property on="Property Node" class="Bool (strict)"(reference=w677, "Value"=w690) -> ()  [unwired: 1 in, 2 out]
                    }
                    frame 3 {
                      w701 = 4 ("Axis")
                      n146 = property on="Theta Multiplier" class="LVObjRef (strict)"() -> ("Value"=w699:refnum<vi>)  [unwired: 2 in, 2 out]
                      n147 = property on="Property Node" class="DigNum (strict)"(reference=w699) -> ("Value"=w708:u32)  [unwired: 1 in, 2 out]
                      n148 = call "Motors Status.vi"("error in"=w709, "VISA in"=w710, "Axis"=w701, "Axis Multiplier"=w708) -> ("error out"=w704:errorcluster, "VISA out"=w705:refnum<visa-resource-name>, "OS"=w715:i32, "Actual Position (mm or deg)"=w707:dbl)  [unwired: 3 in]
                      n149 = call "Motors Datum Position.vi"("error in"=w704, "VISA in"=w705, "Axis"=w701) -> ("error out"=w702:errorcluster, "VISA out"=w703:refnum<visa-resource-name>, "Datum Position (steps)"=w706:string)  [unwired: 5 in]
                      n150 = call "Motors Decipher Status.vi"("OS"=w715) -> ("Status"=w713:string)
                      n151 = property on="Theta (deg)" class="LVObjRef (strict)"() -> ("Value"=w700:refnum<vi>)  [unwired: 2 in, 2 out]
                      n152 = property on="Property Node" class="DigNum (strict)"(reference=w700, "Value"=w707) -> ()  [unwired: 1 in, 2 out]
                      n153 = Equal?(x=w713, y="Idle") -> (x = y?=w712:bool)
                      n154 = property on="Status Theta" class="LVObjRef (strict)"() -> ("Value"=w698:refnum<vi>)  [unwired: 2 in, 2 out]
                      n155 = case shown="True" w712 {
                        tunnel: [TRUE FALSE] -> w711
                        frame False {
                        }
                        frame True {
                        }
                      }
                      n156 = property on="Property Node" class="Str"(reference=w698, "Value"=w713) -> ()  [unwired: 1 in, 2 out]
                      n157 = property on="Theta Moving" class="LVObjRef (strict)"() -> ("Value"=w697:refnum<vi>)  [unwired: 2 in, 2 out]
                      n158 = property on="Property Node" class="Bool (strict)"(reference=w697, "Value"=w711) -> ()  [unwired: 1 in, 2 out]
                    }
                  }
                }
                n159 = Build Array (concatenate)("Limits", w613) -> (w612:string[])
                n160 = Initialize Array("", 0 ("dimension size"), 0 ("dimension size")) -> (w619:string[][])
                n161 = Build Array (concatenate)(w612, w619) -> (w617:string[][])
                n162 = property on="Saved Limits" class="LVObjRef (strict)"() -> ("Value"=w609:refnum<vi>)  [unwired: 2 in, 2 out]
                n163 = property on="Property Node" class="Path"(reference=w609) -> ("Value"=w610:path)  [unwired: 1 in, 2 out]
                n164 = Transpose 2D Array(2D array=w617) -> (transposed array=w616:string[][])
                n165 = call "Motors Position Rewrite.vi"("file path"=w610, "Array of Positions"=w616) -> ()  [unwired: 9 in]
              }
              frame #2 {
                n166 = call <vilib>:"Unset Busy.vi"() -> ()  [unwired: 11 in, 1 out]
                n167 = property on="Property Node" class="Str"(reference=w719, "Value"="Running" ("Status")) -> (reference out=w718:refnum<vi>)  [unwired: 1 in, 1 out]
              }
            }
          }
        }
        n168 = property on="Use Datums Nearest Hard Limits to Reset Origin?" class="LVObjRef (strict)"() -> ("Value"=w143:refnum<vi>)  [unwired: 2 in, 2 out]
        n169 = property on="Property Node" class="Bool (strict)"(reference=w143) -> (reference out=w123:refnum<vi>, "Value"=w241:bool)  [unwired: 1 in, 1 out]
        n170 = case shown="True" w241 {
          tunnel: [w411 w419] -> w250
          tunnel: w249 -> [w411 w421]
          tunnel: [w410 w418] -> w248
          tunnel: w247 -> [w410 w422]
          tunnel: w240 -> [w409 w414]
          tunnel: [w409 w415] -> w168
          tunnel: w123 -> [_ w413]
          frame False {
          }
          frame True {
            n171 = property on="Property Node" class="Bool (strict)"(reference=w413, "Value"=FALSE) -> ()  [unwired: 1 in, 2 out]
            n172 = flat-sequence {
              tunnel: w421 -> [w426]
              tunnel: [w426] -> w420
              tunnel: w414 -> [w424]
              tunnel: [w423] -> w416
              tunnel: w422 -> [w438]
              tunnel: w420 -> [w439]
              tunnel: [w434] -> w419
              tunnel: [w433] -> w418
              tunnel: [w428] -> w417
              tunnel: w416 -> [w428]
              tunnel: w417 -> [w584]
              tunnel: [w583] -> w415
              frame #0 {
                n173 = call <vilib>:"Set Busy.vi"() -> ()  [unwired: 10 in, 2 out]
                n174 = property on="Property Node" class="Str"(reference=w424, "Value"="Finding Datums Nearest Hard Limits\nThis May Take a Few Minutes" ("Status")) -> (reference out=w423:refnum<vi>)  [unwired: 1 in, 1 out]
              }
              frame #1 {
                n175 = property on="Saved Limits" class="LVObjRef (strict)"() -> ("Value"=w427:refnum<vi>)  [unwired: 2 in, 2 out]
                n176 = property on="Property Node" class="Path"(reference=w427) -> ("Value"=w429:path)  [unwired: 1 in, 2 out]
                n177 = call "Motors Find Datums.vi"("error in"=w439, "VISA in"=w438) -> ("error out"=w436:errorcluster, "VISA out"=w437:refnum<visa-resource-name>)
                n178 = call "Motors Position Load.vi"("error in"=w436, "file path"=w429) -> ("error out"=w435:errorcluster, "Positions"=w432:string[][])
                n179 = Delete From Array(array=w432, index (row)=0) -> (array with subset deleted=w430:string[][])  [unwired: 2 in, 1 out]
                n180 = for {
                  shift-right: [w446] -> w434
                  shift-left: w435 -> [w447]
                  shift-right: [w445] -> w433
                  shift-left: w437 -> [w448]
                  tunnel: w430 -> [w444] mode=indexing
                  i -> [w441]
                  n181 = Index Array(array=w444, index=0) -> (element=w443:string)
                  n182 = Fract/Exp String To Number(string=w443) -> (number=w442:dbl)  [unwired: 3 in, 1 out]
                  n183 = case shown="3" w441 {
                    tunnel: w447 -> [w468 w502 w532 w568]
                    tunnel: w448 -> [w469 w503 w533 w569]
                    tunnel: [w462 w495 w524 w561] -> w446
                    tunnel: [w463 w496 w525 w562] -> w445
                    tunnel: w442 -> [w464 w498 w535 w564]
                    frame 0, Default {
                      w452 = u32 1 ("Axis Multiplier")
                      w454 = 1 ("Axis")
                      n184 = property on="Steps to deactivate hard limit after finding datums" class="DigNum (strict)"() -> ("Value"=w460:dbl)  [unwired: 2 in, 2 out]
                      n185 = Negate(x=w460) -> (-x=w455:dbl)
                      n186 = property on="X Multiplier" class="LVObjRef (strict)"() -> ("Value"=w450:refnum<vi>)  [unwired: 2 in, 2 out]
                      n187 = property on="Property Node" class="DigNum (strict)"(reference=w450) -> ("Value"=w453:u32)  [unwired: 1 in, 2 out]
                      n188 = call "Motors Status.vi"("error in"=w468, "VISA in"=w469, "Axis"=w454, "Axis Multiplier"=w453) -> ("error out"=w465:errorcluster, "VISA out"=w466:refnum<visa-resource-name>, "OS"=w473:i32, "Actual Position (mm or deg)"=w467:dbl)  [unwired: 3 in]
                      n189 = call "Motors Position Redefine.vi"("Axis Multiplier"=w452, "Axis"=w454, "error in"=w465, "VISA in"=w466, "Position (mm or deg)"=w464) -> ("error out"=w459:errorcluster, "VISA out"=w456:refnum<visa-resource-name>)  [unwired: 5 in]
                      n190 = call "Motors Decipher Status.vi"("OS"=w473) -> ("Status"=w472:string)
                      n191 = property on="X-Axis (mm)" class="LVObjRef (strict)"() -> ("Value"=w449:refnum<vi>)  [unwired: 2 in, 2 out]
                      n192 = property on="Property Node" class="DigNum (strict)"(reference=w449, "Value"=w467) -> ()  [unwired: 1 in, 2 out]
                      n193 = Equal?(x=w472, y="Idle") -> (x = y?=w470:bool)
                      n194 = property on="Status X" class="LVObjRef (strict)"() -> ("Value"=w451:refnum<vi>)  [unwired: 2 in, 2 out]
                      n195 = property on="Property Node" class="Str"(reference=w451, "Value"=w472) -> ()  [unwired: 1 in, 2 out]
                      n196 = case shown="False" w470 {
                        tunnel: w459 -> [w480 w482]
                        tunnel: [w479 w482] -> w458
                        tunnel: w456 -> [w478 w481]
                        tunnel: [w477 w481] -> w457
                        tunnel: w455 -> [w476 _]
                        tunnel: w454 -> [w475 _]
                        tunnel: w452 -> [w474 _]
                        frame False {
                          n197 = call "Motors Move Relative.vi"("Axis Multiplier"=w474, "Axis"=w475, "error in"=w480, "VISA in"=w478, "Distance (mm)"=w476) -> ("error out"=w479:errorcluster, "VISA out"=w477:refnum<visa-resource-name>)  [unwired: 5 in]
                        }
                        frame True {
                        }
                      }
                      n198 = call "Motors Move Absolute.vi"("Axis Multiplier"=w453, "Axis"=w454, "error in"=w458, "VISA in"=w457, "Position (mm or degree)"=0.0) -> ("error out"=w462:errorcluster, "VISA out"=w463:refnum<visa-resource-name>)  [unwired: 5 in]
                    }
                    frame 1 {
                      w486 = u32 1 ("Axis Multiplier")
                      w488 = 2 ("Axis")
                      n199 = property on="Y Multiplier" class="LVObjRef (strict)"() -> ("Value"=w485:refnum<vi>)  [unwired: 2 in, 2 out]
                      n200 = property on="Steps to deactivate hard limit after finding datums" class="DigNum (strict)"() -> ("Value"=w494:dbl)  [unwired: 2 in, 2 out]
                      n201 = Negate(x=w494) -> (-x=w489:dbl)
                      n202 = property on="Property Node" class="DigNum (strict)"(reference=w485) -> ("Value"=w487:u32)  [unwired: 1 in, 2 out]
                      n203 = call "Motors Status.vi"("error in"=w502, "VISA in"=w503, "Axis"=w488, "Axis Multiplier"=w487) -> ("error out"=w499:errorcluster, "VISA out"=w500:refnum<visa-resource-name>, "OS"=w507:i32, "Actual Position (mm or deg)"=w501:dbl)  [unwired: 3 in]
                      n204 = call "Motors Position Redefine.vi"("Axis Multiplier"=w486, "Axis"=w488, "error in"=w499, "VISA in"=w500, "Position (mm or deg)"=w498) -> ("error out"=w492:errorcluster, "VISA out"=w493:refnum<visa-resource-name>)  [unwired: 5 in]
                      n205 = call "Motors Decipher Status.vi"("OS"=w507) -> ("Status"=w505:string)
                      n206 = property on="Y-Axis (mm)" class="LVObjRef (strict)"() -> ("Value"=w483:refnum<vi>)  [unwired: 2 in, 2 out]
                      n207 = property on="Property Node" class="DigNum (strict)"(reference=w483, "Value"=w501) -> ()  [unwired: 1 in, 2 out]
                      n208 = Equal?(x=w505, y="Idle") -> (x = y?=w504:bool)
                      n209 = property on="Status Y" class="LVObjRef (strict)"() -> ("Value"=w484:refnum<vi>)  [unwired: 2 in, 2 out]
                      n210 = property on="Property Node" class="Str"(reference=w484, "Value"=w505) -> ()  [unwired: 1 in, 2 out]
                      n211 = case shown="False" w504 {
                        tunnel: w493 -> [w514 w515]
                        tunnel: w492 -> [w513 w516]
                        tunnel: [w512 w515] -> w491
                        tunnel: [w511 w516] -> w490
                        tunnel: w489 -> [w510 _]
                        tunnel: w488 -> [w509 _]
                        tunnel: w486 -> [w508 _]
                        frame False {
                          n212 = call "Motors Move Relative.vi"("Axis Multiplier"=w508, "Axis"=w509, "error in"=w513, "VISA in"=w514, "Distance (mm)"=w510) -> ("error out"=w511:errorcluster, "VISA out"=w512:refnum<visa-resource-name>)  [unwired: 5 in]
                        }
                        frame True {
                        }
                      }
                      n213 = call "Motors Move Absolute.vi"("Axis Multiplier"=w487, "Axis"=w488, "error in"=w490, "VISA in"=w491, "Position (mm or degree)"=0.0) -> ("error out"=w495:errorcluster, "VISA out"=w496:refnum<visa-resource-name>)  [unwired: 5 in]
                    }
                    frame 2 {
                      w520 = u32 1 ("Axis Multiplier")
                      w522 = 3 ("Axis")
                      n214 = property on="Z Multiplier" class="LVObjRef (strict)"() -> ("Value"=w518:refnum<vi>)  [unwired: 2 in, 2 out]
                      n215 = property on="Property Node" class="DigNum (strict)"(reference=w518) -> ("Value"=w521:u32)  [unwired: 1 in, 2 out]
                      n216 = call "Motors Status.vi"("error in"=w532, "VISA in"=w533, "Axis"=w522, "Axis Multiplier"=w521) -> ("error out"=w530:errorcluster, "VISA out"=w531:refnum<visa-resource-name>, "OS"=w540:i32, "Actual Position (mm or deg)"=w536:dbl)  [unwired: 3 in]
                      n217 = call "Motors Position Redefine.vi"("Axis Multiplier"=w520, "Axis"=w522, "error in"=w530, "VISA in"=w531, "Position (mm or deg)"=w535) -> ("error out"=w528:errorcluster, "VISA out"=w529:refnum<visa-resource-name>)  [unwired: 5 in]
                      n218 = call "Motors Decipher Status.vi"("OS"=w540) -> ("Status"=w538:string)
                      n219 = property on="Z-Axis (mm)" class="LVObjRef (strict)"() -> ("Value"=w517:refnum<vi>)  [unwired: 2 in, 2 out]
                      n220 = property on="Property Node" class="DigNum (strict)"(reference=w517, "Value"=w536) -> ()  [unwired: 1 in, 2 out]
                      n221 = Equal?(x=w538, y="Idle") -> (x = y?=w537:bool)
                      n222 = property on="Status Z" class="LVObjRef (strict)"() -> ("Value"=w519:refnum<vi>)  [unwired: 2 in, 2 out]
                      n223 = property on="Property Node" class="Str"(reference=w519, "Value"=w538) -> ()  [unwired: 1 in, 2 out]
                      n224 = property on="Steps to deactivate hard limit after finding datums" class="DigNum (strict)"() -> ("Value"=w523:dbl)  [unwired: 2 in, 2 out]
                      n225 = case shown="False" w537 {
                        tunnel: w529 -> [w547 w548]
                        tunnel: w528 -> [w546 w549]
                        tunnel: [w545 w548] -> w527
                        tunnel: [w544 w549] -> w526
                        tunnel: w523 -> [w543 _]
                        tunnel: w522 -> [w542 _]
                        tunnel: w520 -> [w541 _]
                        frame False {
                          n226 = call "Motors Move Relative.vi"("Axis Multiplier"=w541, "Axis"=w542, "error in"=w546, "VISA in"=w547, "Distance (mm)"=w543) -> ("error out"=w544:errorcluster, "VISA out"=w545:refnum<visa-resource-name>)  [unwired: 5 in]
                        }
                        frame True {
                        }
                      }
                      n227 = call "Motors Move Absolute.vi"("Axis Multiplier"=w521, "Axis"=w522, "error in"=w526, "VISA in"=w527, "Position (mm or degree)"=0.0) -> ("error out"=w524:errorcluster, "VISA out"=w525:refnum<visa-resource-name>)  [unwired: 5 in]
                    }
                    frame 3 {
                      w553 = u32 1 ("Axis Multiplier")
                      w555 = 4 ("Axis")
                      n228 = property on="Theta Multiplier" class="LVObjRef (strict)"() -> ("Value"=w551:refnum<vi>)  [unwired: 2 in, 2 out]
                      n229 = property on="Property Node" class="DigNum (strict)"(reference=w551) -> ("Value"=w554:u32)  [unwired: 1 in, 2 out]
                      n230 = call "Motors Status.vi"("error in"=w568, "VISA in"=w569, "Axis"=w555, "Axis Multiplier"=w554) -> ("error out"=w565:errorcluster, "VISA out"=w566:refnum<visa-resource-name>, "OS"=w573:i32, "Actual Position (mm or deg)"=w567:dbl)  [unwired: 3 in]
                      n231 = call "Motors Position Redefine.vi"("Axis Multiplier"=w553, "Axis"=w555, "error in"=w565, "VISA in"=w566, "Position (mm or deg)"=w564) -> ("error out"=w559:errorcluster, "VISA out"=w560:refnum<visa-resource-name>)  [unwired: 5 in]
                      n232 = call "Motors Decipher Status.vi"("OS"=w573) -> ("Status"=w571:string)
                      n233 = property on="Theta (deg)" class="LVObjRef (strict)"() -> ("Value"=w550:refnum<vi>)  [unwired: 2 in, 2 out]
                      n234 = property on="Property Node" class="DigNum (strict)"(reference=w550, "Value"=w567) -> ()  [unwired: 1 in, 2 out]
                      n235 = Equal?(x=w571, y="Idle") -> (x = y?=w570:bool)
                      n236 = property on="Status Theta" class="LVObjRef (strict)"() -> ("Value"=w552:refnum<vi>)  [unwired: 2 in, 2 out]
                      n237 = property on="Property Node" class="Str"(reference=w552, "Value"=w571) -> ()  [unwired: 1 in, 2 out]
                      n238 = case shown="False" w570 {
                        tunnel: w560 -> [w580 w582]
                        tunnel: w559 -> [w579 w581]
                        tunnel: [w578 w582] -> w558
                        tunnel: [w577 w581] -> w557
                        tunnel: "Steps to deactivate hard limit after finding datums" -> [w576 _]
                        tunnel: w555 -> [w575 _]
                        tunnel: w553 -> [w574 _]
                        frame False {
                          n239 = call "Motors Move Relative.vi"("Axis Multiplier"=w574, "Axis"=w575, "error in"=w579, "VISA in"=w580, "Distance (mm)"=w576) -> ("error out"=w577:errorcluster, "VISA out"=w578:refnum<visa-resource-name>)  [unwired: 5 in]
                        }
                        frame True {
                        }
                      }
                      n240 = call "Motors Move Absolute.vi"("Axis Multiplier"=w554, "Axis"=w555, "error in"=w557, "VISA in"=w558, "Position (mm or degree)"=0.0) -> ("error out"=w561:errorcluster, "VISA out"=w562:refnum<visa-resource-name>)  [unwired: 5 in]
                    }
                  }
                }
              }
              frame #2 {
                n241 = call <vilib>:"Unset Busy.vi"() -> ()  [unwired: 11 in, 1 out]
                n242 = property on="Property Node" class="Str"(reference=w584, "Value"="Running" ("Status")) -> (reference out=w583:refnum<vi>)  [unwired: 1 in, 1 out]
              }
            }
          }
        }
        n243 = property on="X Go?" class="LVObjRef (strict)"() -> ("Value"=w142:refnum<vi>)  [unwired: 2 in, 2 out]
        n244 = property on="Property Node" class="Bool (strict)"(reference=w142) -> (reference out=w227:refnum<vi>, "Value"=w239:bool)  [unwired: 1 in, 1 out]
        n245 = case shown="True" w239 {
          tunnel: w248 -> [w1387 w1395]
          tunnel: w250 -> [w1386 w1398]
          tunnel: [w1387 w1396] -> w295
          tunnel: [w1386 w1397] -> w294
          tunnel: w227 -> [_ w1393]
          frame False {
          }
          frame True {
            n246 = property on="Property Node" class="Bool (strict)"(reference=w1393, "Value"=FALSE) -> ()  [unwired: 1 in, 2 out]
            n247 = property on="X Go To" class="LVObjRef (strict)"() -> ("Value"=w1388:refnum<vi>)  [unwired: 2 in, 2 out]
            n248 = property on="X Multiplier" class="LVObjRef (strict)"() -> ("Value"=w1389:refnum<vi>)  [unwired: 2 in, 2 out]
            n249 = property on="Property Node" class="DigNum (strict)"(reference=w1388) -> ("Value"=w1390:dbl)  [unwired: 1 in, 2 out]
            n250 = property on="Property Node" class="DigNum (strict)"(reference=w1389) -> ("Value"=w1391:u32)  [unwired: 1 in, 2 out]
            n251 = call "Motors Move Absolute.vi"("Axis Multiplier"=w1391, "Axis"=u32 1, "error in"=w1398, "VISA in"=w1395, "Position (mm or degree)"=w1390) -> ("error out"=w1397:errorcluster, "VISA out"=w1396:refnum<visa-resource-name>)  [unwired: 5 in]
          }
        }
        n252 = property on="Y Go?" class="LVObjRef (strict)"() -> ("Value"=w141:refnum<vi>)  [unwired: 2 in, 2 out]
        n253 = property on="Property Node" class="Bool (strict)"(reference=w141) -> (reference out=w232:refnum<vi>, "Value"=w233:bool)  [unwired: 1 in, 1 out]
        n254 = case shown="True" w233 {
          tunnel: w295 -> [w1374 w1382]
          tunnel: w294 -> [w1373 w1385]
          tunnel: [w1374 w1383] -> w293
          tunnel: [w1373 w1384] -> w292
          tunnel: w232 -> [_ w1377]
          frame False {
          }
          frame True {
            n255 = property on="Property Node" class="Bool (strict)"(reference=w1377, "Value"=FALSE) -> ()  [unwired: 1 in, 2 out]
            n256 = property on="Y Go To" class="LVObjRef (strict)"() -> ("Value"=w1376:refnum<vi>)  [unwired: 2 in, 2 out]
            n257 = property on="Y Multiplier" class="LVObjRef (strict)"() -> ("Value"=w1375:refnum<vi>)  [unwired: 2 in, 2 out]
            n258 = property on="Property Node" class="DigNum (strict)"(reference=w1375) -> ("Value"=w1380:u32)  [unwired: 1 in, 2 out]
            n259 = property on="Property Node" class="DigNum (strict)"(reference=w1376) -> ("Value"=w1379:dbl)  [unwired: 1 in, 2 out]
            n260 = call "Motors Move Absolute.vi"("Axis Multiplier"=w1380, "Axis"=u32 2, "error in"=w1385, "VISA in"=w1382, "Position (mm or degree)"=w1379) -> ("error out"=w1384:errorcluster, "VISA out"=w1383:refnum<visa-resource-name>)  [unwired: 5 in]
          }
        }
        n261 = property on="Z Go?" class="LVObjRef (strict)"() -> ("Value"=w140:refnum<vi>)  [unwired: 2 in, 2 out]
        n262 = property on="Property Node" class="Bool (strict)"(reference=w140) -> (reference out=w230:refnum<vi>, "Value"=w231:bool)  [unwired: 1 in, 1 out]
        n263 = case shown="True" w231 {
          tunnel: w293 -> [w1361 w1367]
          tunnel: w292 -> [w1360 w1372]
          tunnel: [w1361 w1370] -> w291
          tunnel: [w1360 w1371] -> w290
          tunnel: w230 -> [_ w1364]
          frame False {
          }
          frame True {
            n264 = property on="Property Node" class="Bool (strict)"(reference=w1364, "Value"=FALSE) -> ()  [unwired: 1 in, 2 out]
            n265 = property on="Z Go To" class="LVObjRef (strict)"() -> ("Value"=w1363:refnum<vi>)  [unwired: 2 in, 2 out]
            n266 = property on="Z Multiplier" class="LVObjRef (strict)"() -> ("Value"=w1362:refnum<vi>)  [unwired: 2 in, 2 out]
            n267 = property on="Property Node" class="DigNum (strict)"(reference=w1362) -> ("Value"=w1368:u32)  [unwired: 1 in, 2 out]
            n268 = property on="Property Node" class="DigNum (strict)"(reference=w1363) -> ("Value"=w1366:dbl)  [unwired: 1 in, 2 out]
            n269 = call "Motors Move Absolute.vi"("Axis Multiplier"=w1368, "Axis"=u32 3, "error in"=w1372, "VISA in"=w1367, "Position (mm or degree)"=w1366) -> ("error out"=w1371:errorcluster, "VISA out"=w1370:refnum<visa-resource-name>)  [unwired: 5 in]
          }
        }
        n270 = property on="Theta Go?" class="LVObjRef (strict)"() -> ("Value"=w139:refnum<vi>)  [unwired: 2 in, 2 out]
        n271 = property on="Property Node" class="Bool (strict)"(reference=w139) -> (reference out=w228:refnum<vi>, "Value"=w229:bool)  [unwired: 1 in, 1 out]
        n272 = case shown="True" w229 {
          tunnel: w291 -> [w1347 w1356]
          tunnel: w290 -> [w1348 w1359]
          tunnel: [w1348 w1358] -> w288
          tunnel: [w1347 w1357] -> w289
          tunnel: w228 -> [_ w1351]
          frame False {
          }
          frame True {
            n273 = property on="Property Node" class="Bool (strict)"(reference=w1351, "Value"=FALSE) -> ()  [unwired: 1 in, 2 out]
            n274 = property on="Theta Multiplier" class="LVObjRef (strict)"() -> ("Value"=w1349:refnum<vi>)  [unwired: 2 in, 2 out]
            n275 = property on="Theta Go To" class="LVObjRef (strict)"() -> ("Value"=w1350:refnum<vi>)  [unwired: 2 in, 2 out]
            n276 = property on="Property Node" class="DigNum (strict)"(reference=w1349) -> ("Value"=w1354:u32)  [unwired: 1 in, 2 out]
            n277 = property on="Property Node" class="DigNum (strict)"(reference=w1350) -> ("Value"=w1353:dbl)  [unwired: 1 in, 2 out]
            n278 = call "Motors Move Absolute.vi"("Axis Multiplier"=w1354, "Axis"=u32 4, "error in"=w1359, "VISA in"=w1356, "Position (mm or degree)"=w1353) -> ("error out"=w1358:errorcluster, "VISA out"=w1357:refnum<visa-resource-name>)  [unwired: 5 in]
          }
        }
        n279 = property on="x+?" class="LVObjRef (strict)"() -> ("Value"=w137:refnum<vi>)  [unwired: 2 in, 2 out]
        n280 = property on="x-?" class="LVObjRef (strict)"() -> ("Value"=w136:refnum<vi>)  [unwired: 2 in, 2 out]
        n281 = property on="Property Node" class="Bool (strict)"(reference=w137) -> (reference out=w225:refnum<vi>, "Value"=w260:bool)  [unwired: 1 in, 1 out]
        n282 = property on="Property Node" class="Bool (strict)"(reference=w136) -> (reference out=w226:refnum<vi>, "Value"=w259:bool)  [unwired: 1 in, 1 out]
        n283 = property on="Jog-Mode" class="LVObjRef (strict)"() -> ("Value"=w138:refnum<vi>)  [unwired: 2 in, 2 out]
        n284 = property on="Property Node" class="Bool (strict)"(reference=w138) -> ("Value"=w185:bool)  [unwired: 1 in, 2 out]
        n285 = Or(x=w260, y=w259) -> (x .or. y?=w287:bool)
        n286 = case shown="True" w287 {
          tunnel: w289 -> [w1259 w1269]
          tunnel: w288 -> [w1258 w1268]
          tunnel: w185 -> [_ w1270]
          tunnel: [w1259 w1266] -> w286
          tunnel: [w1258 w1265] -> w285
          tunnel: w259 -> [_ w1267]
          tunnel: w226 -> [_ w1262]
          tunnel: w225 -> [_ w1261]
          frame False {
          }
          frame True {
            n287 = property on="X Multiplier" class="LVObjRef (strict)"() -> ("Value"=w1260:refnum<vi>)  [unwired: 2 in, 2 out]
            n288 = flat-sequence {
              tunnel: w1270 -> [w1277]
              tunnel: w1269 -> [w1276]
              tunnel: w1268 -> [w1275]
              tunnel: w1267 -> [w1274]
              tunnel: [w1273] -> w1264
              tunnel: [w1272] -> w1263
              tunnel: w1260 -> [w1271]
              tunnel: [w1345] -> w1265
              tunnel: [w1346] -> w1266
              tunnel: w1264 -> [w1346]
              tunnel: w1263 -> [w1345]
              tunnel: w1262 -> [w1342]
              tunnel: w1261 -> [w1341]
              frame #0 {
                n289 = case shown="True" w1277 {
                  tunnel: w1276 -> [w1286 w1312]
                  tunnel: w1275 -> [w1282 w1315]
                  tunnel: w1274 -> [w1285 w1320]
                  tunnel: [w1284 w1317] -> w1273
                  tunnel: [w1283 w1316] -> w1272
                  tunnel: w1271 -> [w1279 w1307]
                  frame False {
                    n290 = property on="X Moving" class="LVObjRef (strict)"() -> ("Value"=w1278:refnum<vi>)  [unwired: 2 in, 2 out]
                    n291 = property on="Property Node" class="Bool (strict)"(reference=w1278) -> (reference out=w1280:refnum<vi>, "Value"=w1281:bool)  [unwired: 1 in, 1 out]
                    n292 = case shown="False" w1281 {
                      tunnel: w1286 -> [w1294 w1305]
                      tunnel: w1282 -> [w1299 w1304]
                      tunnel: w1285 -> [w1298 _]
                      tunnel: [w1296 w1305] -> w1284
                      tunnel: [w1297 w1304] -> w1283
                      tunnel: w1280 -> [w1290 _]
                      tunnel: w1279 -> [w1288 _]
                      frame False {
                        n293 = property on="Delta X (mm)" class="LVObjRef (strict)"() -> ("Value"=w1287:refnum<vi>)  [unwired: 2 in, 2 out]
                        n294 = property on="Property Node" class="DigNum (strict)"(reference=w1287) -> ("Value"=w1289:dbl)  [unwired: 1 in, 2 out]
                        n295 = property on="Property Node" class="Bool (strict)"(reference=w1290, "Value"=TRUE ("X Moving")) -> ()  [unwired: 1 in, 2 out]
                        n296 = property on="Property Node" class="DigNum (strict)"(reference=w1288) -> ("Value"=w1292:u32)  [unwired: 1 in, 2 out]
                        n297 = case shown="True" w1298 {
                          tunnel: w1289 -> [w1300 w1302]
                          tunnel: [w1300 w1301] -> w1295
                          frame False {
                          }
                          frame True {
                            n298 = Multiply(x=w1302, y=-1.0) -> (x*y=w1301:dbl)
                          }
                        }
                        n299 = call "Motors Move Relative.vi"("Axis Multiplier"=w1292, "Axis"=1, "error in"=w1299, "VISA in"=w1294, "Distance (mm)"=w1295) -> ("error out"=w1297:errorcluster, "VISA out"=w1296:refnum<visa-resource-name>)  [unwired: 5 in]
                      }
                      frame True {
                      }
                    }
                  }
                  frame True {
                    w1309 = 1 ("Axis")
                    n300 = property on="Property Node" class="DigNum (strict)"(reference=w1307) -> ("Value"=w1310:u32)  [unwired: 1 in, 2 out]
                    n301 = property on="X Speed (mm/s)" class="LVObjRef (strict)"() -> ("Value"=w1306:refnum<vi>)  [unwired: 2 in, 2 out]
                    n302 = property on="Property Node" class="DigNum (strict)"(reference=w1306) -> ("Value"=w1308:dbl)  [unwired: 1 in, 2 out]
                    n303 = case shown="True" w1320 {
                      tunnel: w1308 -> [w1337 w1339]
                      tunnel: [w1337 w1338] -> w1313
                      frame False {
                      }
                      frame True {
                        n304 = Multiply(x=w1339, y=-1.0) -> (x*y=w1338:dbl)
                      }
                    }
                    n305 = call "Motors Move Constant Velocity.vi"("Axis Multiplier"=w1310, "Axis"=w1309, "error in"=w1315, "VISA in"=w1312, "Speed (mm/s)"=w1313) -> ("error out"=w1314:errorcluster, "VISA out"=w1311:refnum<visa-resource-name>)  [unwired: 5 in]
                    n306 = while {
                      tunnel: w1311 -> [w1326]
                      tunnel: [w1328] -> w1319
                      tunnel: w1314 -> [w1329]
                      tunnel: [w1327] -> w1318
                      tunnel: w1310 -> [w1325]
                      stop <- w1334 continue-if-true
                      n307 = property on="x+" class="LVObjRef (strict)"() -> ("Value"=w1321:refnum<vi>)  [unwired: 2 in, 2 out]
                      n308 = property on="x-" class="LVObjRef (strict)"() -> ("Value"=w1322:refnum<vi>)  [unwired: 2 in, 2 out]
                      n309 = property on="Property Node" class="Bool (strict)"(reference=w1321) -> ("Value"=w1335:bool)  [unwired: 1 in, 2 out]
                      n310 = property on="Property Node" class="Bool (strict)"(reference=w1322) -> ("Value"=w1336:bool)  [unwired: 1 in, 2 out]
                      n311 = call "Motors Status.vi"("error in"=w1329, "VISA in"=w1326, "Axis"=1, "Axis Multiplier"=w1325) -> ("error out"=w1327:errorcluster, "VISA out"=w1328:refnum<visa-resource-name>, "OS"=w1332:i32, "Actual Position (mm or deg)"=w1330:dbl)  [unwired: 3 in]
                      n312 = Or(x=w1335, y=w1336) -> (x .or. y?=w1334:bool)
                      n313 = call "Motors Decipher Status.vi"("OS"=w1332) -> ("Status"=w1331:string)
                      n314 = property on="X-Axis (mm)" class="LVObjRef (strict)"() -> ("Value"=w1324:refnum<vi>)  [unwired: 2 in, 2 out]
                      n315 = property on="Property Node" class="DigNum (strict)"(reference=w1324, "Value"=w1330) -> ()  [unwired: 1 in, 2 out]
                      n316 = property on="Status X" class="LVObjRef (strict)"() -> ("Value"=w1323:refnum<vi>)  [unwired: 2 in, 2 out]
                      n317 = property on="Property Node" class="Str"(reference=w1323, "Value"=w1331) -> ()  [unwired: 1 in, 2 out]
                    }
                    n318 = call "Motors Stop.vi"("error in"=w1318, "Axis"=w1309, "VISA in"=w1319) -> ("error out"=w1316:errorcluster, "VISA out"=w1317:refnum<visa-resource-name>)
                  }
                }
              }
              frame #1 {
                n319 = property on="Property Node" class="Bool (strict)"(reference=w1341, "Value"=FALSE) -> ()  [unwired: 1 in, 2 out]
                n320 = property on="Property Node" class="Bool (strict)"(reference=w1342, "Value"=FALSE) -> ()  [unwired: 1 in, 2 out]
              }
            }
          }
        }
        n321 = property on="y+?" class="LVObjRef (strict)"() -> ("Value"=w134:refnum<vi>)  [unwired: 2 in, 2 out]
        n322 = property on="y-?" class="LVObjRef (strict)"() -> ("Value"=w133:refnum<vi>)  [unwired: 2 in, 2 out]
        n323 = property on="Property Node" class="Bool (strict)"(reference=w134) -> (reference out=w183:refnum<vi>, "Value"=w258:bool)  [unwired: 1 in, 1 out]
        n324 = property on="Property Node" class="Bool (strict)"(reference=w133) -> (reference out=w182:refnum<vi>, "Value"=w257:bool)  [unwired: 1 in, 1 out]
        n325 = property on="Jog-Mode" class="LVObjRef (strict)"() -> ("Value"=w135:refnum<vi>)  [unwired: 2 in, 2 out]
        n326 = property on="Property Node" class="Bool (strict)"(reference=w135) -> ("Value"=w184:bool)  [unwired: 1 in, 2 out]
        n327 = Or(x=w258, y=w257) -> (x .or. y?=w284:bool)
        n328 = case shown="True" w284 {
          tunnel: w286 -> [w1171 w1180]
          tunnel: w285 -> [w1170 w1179]
          tunnel: w184 -> [_ w1181]
          tunnel: [w1171 w1178] -> w283
          tunnel: [w1170 w1177] -> w282
          tunnel: w257 -> [_ w1176]
          tunnel: w183 -> [_ w1173]
          tunnel: w182 -> [_ w1172]
          frame False {
          }
          frame True {
            n329 = flat-sequence {
              tunnel: w1181 -> [w1188]
              tunnel: w1180 -> [w1187]
              tunnel: w1179 -> [w1186]
              tunnel: w1176 -> [w1183]
              tunnel: [w1185] -> w1175
              tunnel: [w1184] -> w1174
              tunnel: [w1256] -> w1177
              tunnel: [w1257] -> w1178
              tunnel: w1175 -> [w1257]
              tunnel: w1174 -> [w1256]
              tunnel: w1173 -> [w1253]
              tunnel: w1172 -> [w1252]
              frame #0 {
                n330 = property on="Y Multiplier" class="LVObjRef (strict)"() -> ("Value"=w1182:refnum<vi>)  [unwired: 2 in, 2 out]
                n331 = case shown="True" w1188 {
                  tunnel: w1187 -> [w1197 w1223]
                  tunnel: w1186 -> [w1196 w1226]
                  tunnel: [w1195 w1229] -> w1185
                  tunnel: [w1194 w1228] -> w1184
                  tunnel: w1183 -> [w1193 w1227]
                  tunnel: w1182 -> [w1191 w1218]
                  frame False {
                    n332 = property on="Y Moving" class="LVObjRef (strict)"() -> ("Value"=w1189:refnum<vi>)  [unwired: 2 in, 2 out]
                    n333 = property on="Property Node" class="Bool (strict)"(reference=w1189) -> (reference out=w1190:refnum<vi>, "Value"=w1192:bool)  [unwired: 1 in, 1 out]
                    n334 = case shown="False" w1192 {
                      tunnel: w1197 -> [w1206 w1216]
                      tunnel: w1196 -> [w1210 w1215]
                      tunnel: [w1207 w1216] -> w1195
                      tunnel: [w1209 w1215] -> w1194
                      tunnel: w1193 -> [w1208 _]
                      tunnel: w1191 -> [w1201 _]
                      tunnel: w1190 -> [w1200 _]
                      frame False {
                        n335 = property on="Delta Y (mm)" class="LVObjRef (strict)"() -> ("Value"=w1198:refnum<vi>)  [unwired: 2 in, 2 out]
                        n336 = property on="Property Node" class="DigNum (strict)"(reference=w1198) -> ("Value"=w1199:dbl)  [unwired: 1 in, 2 out]
                        n337 = property on="Property Node" class="Bool (strict)"(reference=w1200, "Value"=TRUE ("Y Moving")) -> ()  [unwired: 1 in, 2 out]
                        n338 = property on="Property Node" class="DigNum (strict)"(reference=w1201) -> ("Value"=w1203:u32)  [unwired: 1 in, 2 out]
                        n339 = case shown="True" w1208 {
                          tunnel: w1199 -> [w1211 w1213]
                          tunnel: [w1211 w1212] -> w1205
                          frame False {
                          }
                          frame True {
                            n340 = Multiply(x=w1213, y=-1.0) -> (x*y=w1212:dbl)
                          }
                        }
                        n341 = call "Motors Move Relative.vi"("Axis Multiplier"=w1203, "Axis"=2, "error in"=w1210, "VISA in"=w1206, "Distance (mm)"=w1205) -> ("error out"=w1209:errorcluster, "VISA out"=w1207:refnum<visa-resource-name>)  [unwired: 5 in]
                      }
                      frame True {
                      }
                    }
                  }
                  frame True {
                    w1220 = 2 ("Axis")
                    n342 = property on="Property Node" class="DigNum (strict)"(reference=w1218) -> ("Value"=w1221:u32)  [unwired: 1 in, 2 out]
                    n343 = property on="Y Speed (mm/s)" class="LVObjRef (strict)"() -> ("Value"=w1217:refnum<vi>)  [unwired: 2 in, 2 out]
                    n344 = property on="Property Node" class="DigNum (strict)"(reference=w1217) -> ("Value"=w1219:dbl)  [unwired: 1 in, 2 out]
                    n345 = case shown="True" w1227 {
                      tunnel: w1219 -> [w1248 w1250]
                      tunnel: [w1248 w1249] -> w1224
                      frame False {
                      }
                      frame True {
                        n346 = Multiply(x=w1250, y=-1.0) -> (x*y=w1249:dbl)
                      }
                    }
                    n347 = call "Motors Move Constant Velocity.vi"("Axis Multiplier"=w1221, "Axis"=w1220, "error in"=w1226, "VISA in"=w1223, "Speed (mm/s)"=w1224) -> ("error out"=w1225:errorcluster, "VISA out"=w1222:refnum<visa-resource-name>)  [unwired: 5 in]
                    n348 = while {
                      tunnel: w1222 -> [w1238]
                      tunnel: [w1237] -> w1231
                      tunnel: w1225 -> [w1240]
                      tunnel: [w1239] -> w1230
                      tunnel: w1221 -> [w1236]
                      stop <- w1247 continue-if-true
                      n349 = property on="y+" class="LVObjRef (strict)"() -> ("Value"=w1232:refnum<vi>)  [unwired: 2 in, 2 out]
                      n350 = property on="y-" class="LVObjRef (strict)"() -> ("Value"=w1233:refnum<vi>)  [unwired: 2 in, 2 out]
                      n351 = property on="Property Node" class="Bool (strict)"(reference=w1232) -> ("Value"=w1246:bool)  [unwired: 1 in, 2 out]
                      n352 = property on="Property Node" class="Bool (strict)"(reference=w1233) -> ("Value"=w1245:bool)  [unwired: 1 in, 2 out]
                      n353 = call "Motors Status.vi"("error in"=w1240, "VISA in"=w1238, "Axis"=2, "Axis Multiplier"=w1236) -> ("error out"=w1239:errorcluster, "VISA out"=w1237:refnum<visa-resource-name>, "OS"=w1242:i32, "Actual Position (mm or deg)"=w1243:dbl)  [unwired: 3 in]
                      n354 = Or(x=w1246, y=w1245) -> (x .or. y?=w1247:bool)
                      n355 = call "Motors Decipher Status.vi"("OS"=w1242) -> ("Status"=w1241:string)
                      n356 = property on="Y-Axis (mm)" class="LVObjRef (strict)"() -> ("Value"=w1235:refnum<vi>)  [unwired: 2 in, 2 out]
                      n357 = property on="Status Y" class="LVObjRef (strict)"() -> ("Value"=w1234:refnum<vi>)  [unwired: 2 in, 2 out]
                      n358 = property on="Property Node" class="Str"(reference=w1234, "Value"=w1241) -> ()  [unwired: 1 in, 2 out]
                      n359 = property on="Property Node" class="DigNum (strict)"(reference=w1235, "Value"=w1243) -> ()  [unwired: 1 in, 2 out]
                    }
                    n360 = call "Motors Stop.vi"("error in"=w1230, "Axis"=w1220, "VISA in"=w1231) -> ("error out"=w1228:errorcluster, "VISA out"=w1229:refnum<visa-resource-name>)
                  }
                }
              }
              frame #1 {
                n361 = property on="Property Node" class="Bool (strict)"(reference=w1253, "Value"=FALSE) -> ()  [unwired: 1 in, 2 out]
                n362 = property on="Property Node" class="Bool (strict)"(reference=w1252, "Value"=FALSE) -> ()  [unwired: 1 in, 2 out]
              }
            }
          }
        }
        n363 = property on="z-?" class="LVObjRef (strict)"() -> ("Value"=w130:refnum<vi>)  [unwired: 2 in, 2 out]
        n364 = property on="z+?" class="LVObjRef (strict)"() -> ("Value"=w131:refnum<vi>)  [unwired: 2 in, 2 out]
        n365 = property on="Property Node" class="Bool (strict)"(reference=w130) -> (reference out=w224:refnum<vi>, "Value"=w256:bool)  [unwired: 1 in, 1 out]
        n366 = property on="Property Node" class="Bool (strict)"(reference=w131) -> (reference out=w223:refnum<vi>, "Value"=w255:bool)  [unwired: 1 in, 1 out]
        n367 = property on="Jog-Mode" class="LVObjRef (strict)"() -> ("Value"=w132:refnum<vi>)  [unwired: 2 in, 2 out]
        n368 = property on="Property Node" class="Bool (strict)"(reference=w132) -> ("Value"=w181:bool)  [unwired: 1 in, 2 out]
        n369 = Or(x=w255, y=w256) -> (x .or. y?=w281:bool)
        n370 = case shown="True" w281 {
          tunnel: w283 -> [w1079 w1089]
          tunnel: w282 -> [w1078 w1083]
          tunnel: w181 -> [_ w1090]
          tunnel: [w1079 w1088] -> w278
          tunnel: [w1078 w1087] -> w279
          tunnel: w256 -> [_ w1086]
          tunnel: w224 -> [_ w1082]
          tunnel: w224 -> [_ w1081]
          tunnel: w223 -> [_ w1080]
          frame False {
          }
          frame True {
            n371 = flat-sequence {
              tunnel: w1090 -> [w1098]
              tunnel: w1089 -> [w1097]
              tunnel: w1086 -> [w1094]
              tunnel: [w1096] -> w1085
              tunnel: [w1095] -> w1084
              tunnel: w1083 -> [w1093]
              tunnel: w1082 -> [w1092]
              tunnel: [w1168] -> w1087
              tunnel: [w1169] -> w1088
              tunnel: w1085 -> [w1169]
              tunnel: w1084 -> [w1168]
              tunnel: w1081 -> [w1165]
              tunnel: w1080 -> [w1164]
              frame #0 {
                n372 = property on="Z Multiplier" class="LVObjRef (strict)"() -> ("Value"=w1091:refnum<vi>)  [unwired: 2 in, 2 out]
                n373 = case shown="False" w1098 {
                  tunnel: w1097 -> [w1107 w1135]
                  tunnel: w1093 -> [w1106 w1138]
                  tunnel: [w1105 w1141] -> w1096
                  tunnel: [w1104 w1140] -> w1095
                  tunnel: w1094 -> [w1103 w1130]
                  tunnel: w1093 -> [_ w1132]
                  tunnel: w1092 -> [_ w1129]
                  tunnel: w1091 -> [w1100 w1128]
                  frame False {
                    n374 = property on="Z Moving" class="LVObjRef (strict)"() -> ("Value"=w1099:refnum<vi>)  [unwired: 2 in, 2 out]
                    n375 = property on="Property Node" class="Bool (strict)"(reference=w1099) -> (reference out=w1101:refnum<vi>, "Value"=w1102:bool)  [unwired: 1 in, 1 out]
                    n376 = case shown="False" w1102 {
                      tunnel: w1107 -> [w1113 w1126]
                      tunnel: w1106 -> [w1120 w1125]
                      tunnel: [w1114 w1126] -> w1105
                      tunnel: [w1119 w1125] -> w1104
                      tunnel: w1103 -> [w1118 _]
                      tunnel: w1101 -> [w1110 _]
                      tunnel: w1100 -> [w1109 _]
                      frame False {
                        n377 = property on="Delta Z (mm)" class="LVObjRef (strict)"() -> ("Value"=w1108:refnum<vi>)  [unwired: 2 in, 2 out]
                        n378 = property on="Property Node" class="DigNum (strict)"(reference=w1108) -> ("Value"=w1111:dbl)  [unwired: 1 in, 2 out]
                        n379 = property on="Property Node" class="Bool (strict)"(reference=w1110, "Value"=TRUE ("Z Moving")) -> ()  [unwired: 1 in, 2 out]
                        n380 = property on="Property Node" class="DigNum (strict)"(reference=w1109) -> ("Value"=w1116:u32)  [unwired: 1 in, 2 out]
                        n381 = case shown="True" w1118 {
                          tunnel: w1111 -> [w1121 w1123]
                          tunnel: [w1121 w1122] -> w1115
                          frame False {
                          }
                          frame True {
                            n382 = Multiply(x=w1123, y=-1.0) -> (x*y=w1122:dbl)
                          }
                        }
                        n383 = call "Motors Move Relative.vi"("Axis Multiplier"=w1116, "Axis"=3, "error in"=w1120, "VISA in"=w1113, "Distance (mm)"=w1115) -> ("error out"=w1119:errorcluster, "VISA out"=w1114:refnum<visa-resource-name>)  [unwired: 5 in]
                      }
                      frame True {
                      }
                    }
                  }
                  frame True {
                    w1137 = 3 ("Axis")
                    n384 = property on="Property Node" class="DigNum (strict)"(reference=w1128) -> ("Value"=w1133:u32)  [unwired: 1 in, 2 out]
                    n385 = property on="Z Speed (mm/s)" class="LVObjRef (strict)"() -> ("Value"=w1127:refnum<vi>)  [unwired: 2 in, 2 out]
                    n386 = property on="Property Node" class="DigNum (strict)"(reference=w1127, error in=w1132) -> ("Value"=w1131:dbl)  [unwired: 2 out]
                    n387 = case shown="True" w1130 {
                      tunnel: w1131 -> [w1160 w1162]
                      tunnel: [w1160 w1161] -> w1136
                      frame False {
                      }
                      frame True {
                        n388 = Multiply(x=w1162, y=-1.0) -> (x*y=w1161:dbl)
                      }
                    }
                    n389 = call "Motors Move Constant Velocity.vi"("Axis Multiplier"=w1133, "Axis"=w1137, "error in"=w1138, "VISA in"=w1135, "Speed (mm/s)"=w1136) -> ("error out"=w1139:errorcluster, "VISA out"=w1134:refnum<visa-resource-name>)  [unwired: 5 in]
                    n390 = while {
                      tunnel: w1134 -> [w1150]
                      tunnel: [w1149] -> w1143
                      tunnel: w1139 -> [w1152]
                      tunnel: [w1151] -> w1142
                      tunnel: w1133 -> [w1148]
                      tunnel: w1129 -> [_]
                      stop <- w1159 continue-if-true
                      n391 = property on="z+" class="LVObjRef (strict)"() -> ("Value"=w1146:refnum<vi>)  [unwired: 2 in, 2 out]
                      n392 = property on="z-" class="LVObjRef (strict)"() -> ("Value"=w1145:refnum<vi>)  [unwired: 2 in, 2 out]
                      n393 = property on="Property Node" class="Bool (strict)"(reference=w1146) -> ("Value"=w1158:bool)  [unwired: 1 in, 2 out]
                      n394 = property on="Property Node" class="Bool (strict)"(reference=w1145) -> ("Value"=w1157:bool)  [unwired: 1 in, 2 out]
                      n395 = call "Motors Status.vi"("error in"=w1152, "VISA in"=w1150, "Axis"=3, "Axis Multiplier"=w1148) -> ("error out"=w1151:errorcluster, "VISA out"=w1149:refnum<visa-resource-name>, "OS"=w1154:i32, "Actual Position (mm or deg)"=w1155:dbl)  [unwired: 3 in]
                      n396 = Or(x=w1158, y=w1157) -> (x .or. y?=w1159:bool)
                      n397 = call "Motors Decipher Status.vi"("OS"=w1154) -> ("Status"=w1153:string)
                      n398 = property on="Z-Axis (mm)" class="LVObjRef (strict)"() -> ("Value"=w1144:refnum<vi>)  [unwired: 2 in, 2 out]
                      n399 = property on="Status Z" class="LVObjRef (strict)"() -> ("Value"=w1147:refnum<vi>)  [unwired: 2 in, 2 out]
                      n400 = property on="Property Node" class="Str"(reference=w1147, "Value"=w1153) -> ()  [unwired: 1 in, 2 out]
                      n401 = property on="Property Node" class="DigNum (strict)"(reference=w1144, "Value"=w1155) -> ()  [unwired: 1 in, 2 out]
                    }
                    n402 = call "Motors Stop.vi"("error in"=w1142, "Axis"=w1137, "VISA in"=w1143) -> ("error out"=w1140:errorcluster, "VISA out"=w1141:refnum<visa-resource-name>)
                  }
                }
              }
              frame #1 {
                n403 = property on="Property Node" class="Bool (strict)"(reference=w1165, "Value"=FALSE) -> ()  [unwired: 1 in, 2 out]
                n404 = property on="Property Node" class="Bool (strict)"(reference=w1164, "Value"=FALSE) -> ()  [unwired: 1 in, 2 out]
              }
            }
          }
        }
        n405 = property on="theta-?" class="LVObjRef (strict)"() -> ("Value"=w127:refnum<vi>)  [unwired: 2 in, 2 out]
        n406 = property on="theta+?" class="LVObjRef (strict)"() -> ("Value"=w128:refnum<vi>)  [unwired: 2 in, 2 out]
        n407 = property on="Property Node" class="Bool (strict)"(reference=w128) -> (reference out=w179:refnum<vi>, "Value"=w254:bool)  [unwired: 1 in, 1 out]
        n408 = property on="Property Node" class="Bool (strict)"(reference=w127) -> (reference out=w180:refnum<vi>, "Value"=w253:bool)  [unwired: 1 in, 1 out]
        n409 = property on="Jog-Mode" class="LVObjRef (strict)"() -> ("Value"=w129:refnum<vi>)  [unwired: 2 in, 2 out]
        n410 = property on="Property Node" class="Bool (strict)"(reference=w129) -> ("Value"=w186:bool)  [unwired: 1 in, 2 out]
        n411 = Or(x=w254, y=w253) -> (x .or. y?=w280:bool)
        n412 = case shown="True" w280 {
          tunnel: w278 -> [w991 w1000]
          tunnel: w279 -> [w990 w999]
          tunnel: w186 -> [_ w1001]
          tunnel: [w991 w998] -> w277
          tunnel: [w990 w997] -> w270
          tunnel: w253 -> [_ w996]
          tunnel: w180 -> [_ w993]
          tunnel: w179 -> [_ w992]
          frame False {
          }
          frame True {
            n413 = flat-sequence {
              tunnel: w1001 -> [w1008]
              tunnel: w1000 -> [w1007]
              tunnel: w999 -> [w1006]
              tunnel: w996 -> [w1003]
              tunnel: [w1005] -> w995
              tunnel: [w1004] -> w994
              tunnel: [w1076] -> w997
              tunnel: [w1077] -> w998
              tunnel: w995 -> [w1077]
              tunnel: w994 -> [w1076]
              tunnel: w993 -> [w1073]
              tunnel: w992 -> [w1072]
              frame #0 {
                n414 = property on="Theta Multiplier" class="LVObjRef (strict)"() -> ("Value"=w1002:refnum<vi>)  [unwired: 2 in, 2 out]
                n415 = case shown="True" w1008 {
                  tunnel: w1007 -> [w1017 w1044]
                  tunnel: w1006 -> [w1016 w1045]
                  tunnel: [w1015 w1049] -> w1005
                  tunnel: [w1014 w1048] -> w1004
                  tunnel: w1003 -> [w1013 w1047]
                  tunnel: w1002 -> [w1011 w1039]
                  frame False {
                    n416 = property on="Theta Moving" class="LVObjRef (strict)"() -> ("Value"=w1009:refnum<vi>)  [unwired: 2 in, 2 out]
                    n417 = property on="Property Node" class="Bool (strict)"(reference=w1009) -> (reference out=w1010:refnum<vi>, "Value"=w1012:bool)  [unwired: 1 in, 1 out]
                    n418 = case shown="False" w1012 {
                      tunnel: w1017 -> [w1024 w1036]
                      tunnel: w1016 -> [w1030 w1035]
                      tunnel: [w1025 w1036] -> w1015
                      tunnel: [w1029 w1035] -> w1014
                      tunnel: w1013 -> [w1028 _]
                      tunnel: w1011 -> [w1021 _]
                      tunnel: w1010 -> [w1020 _]
                      frame False {
                        n419 = property on="Delta Theta (deg)" class="LVObjRef (strict)"() -> ("Value"=w1018:refnum<vi>)  [unwired: 2 in, 2 out]
                        n420 = property on="Property Node" class="DigNum (strict)"(reference=w1018) -> ("Value"=w1019:dbl)  [unwired: 1 in, 2 out]
                        n421 = property on="Property Node" class="Bool (strict)"(reference=w1020, "Value"=TRUE ("Theta Moving")) -> ()  [unwired: 1 in, 2 out]
                        n422 = property on="Property Node" class="DigNum (strict)"(reference=w1021) -> ("Value"=w1027:u32)  [unwired: 1 in, 2 out]
                        n423 = case shown="True" w1028 {
                          tunnel: w1019 -> [w1031 w1033]
                          tunnel: [w1031 w1032] -> w1023
                          frame False {
                          }
                          frame True {
                            n424 = Multiply(x=w1033, y=-1.0) -> (x*y=w1032:dbl)
                          }
                        }
                        n425 = call "Motors Move Relative.vi"("Axis Multiplier"=w1027, "Axis"=4, "error in"=w1030, "VISA in"=w1024, "Distance (mm)"=w1023) -> ("error out"=w1029:errorcluster, "VISA out"=w1025:refnum<visa-resource-name>)  [unwired: 5 in]
                      }
                      frame True {
                      }
                    }
                  }
                  frame True {
                    w1042 = 4 ("Axis")
                    n426 = property on="Property Node" class="DigNum (strict)"(reference=w1039) -> ("Value"=w1041:u32)  [unwired: 1 in, 2 out]
                    n427 = property on="Theta Speed (deg/s)" class="LVObjRef (strict)"() -> ("Value"=w1037:refnum<vi>)  [unwired: 2 in, 2 out]
                    n428 = property on="Property Node" class="DigNum (strict)"(reference=w1037) -> ("Value"=w1038:dbl)  [unwired: 1 in, 2 out]
                    n429 = case shown="True" w1047 {
                      tunnel: w1038 -> [w1068 w1070]
                      tunnel: [w1068 w1069] -> w1040
                      frame False {
                      }
                      frame True {
                        n430 = Multiply(x=w1070, y=-1.0) -> (x*y=w1069:dbl)
                      }
                    }
                    n431 = call "Motors Move Constant Velocity.vi"("Axis Multiplier"=w1041, "Axis"=w1042, "error in"=w1045, "VISA in"=w1044, "Speed (mm/s)"=w1040) -> ("error out"=w1046:errorcluster, "VISA out"=w1043:refnum<visa-resource-name>)  [unwired: 5 in]
                    n432 = while {
                      tunnel: w1043 -> [w1058]
                      tunnel: [w1057] -> w1051
                      tunnel: w1046 -> [w1060]
                      tunnel: [w1059] -> w1050
                      tunnel: w1041 -> [w1056]
                      stop <- w1067 continue-if-true
                      n433 = property on="theta+" class="LVObjRef (strict)"() -> ("Value"=w1053:refnum<vi>)  [unwired: 2 in, 2 out]
                      n434 = property on="theta-" class="LVObjRef (strict)"() -> ("Value"=w1054:refnum<vi>)  [unwired: 2 in, 2 out]
                      n435 = property on="Property Node" class="Bool (strict)"(reference=w1053) -> ("Value"=w1066:bool)  [unwired: 1 in, 2 out]
                      n436 = property on="Property Node" class="Bool (strict)"(reference=w1054) -> ("Value"=w1065:bool)  [unwired: 1 in, 2 out]
                      n437 = call "Motors Status.vi"("error in"=w1060, "VISA in"=w1058, "Axis"=4, "Axis Multiplier"=w1056) -> ("error out"=w1059:errorcluster, "VISA out"=w1057:refnum<visa-resource-name>, "OS"=w1062:i32, "Actual Position (mm or deg)"=w1063:dbl)  [unwired: 3 in]
                      n438 = Or(x=w1066, y=w1065) -> (x .or. y?=w1067:bool)
                      n439 = call "Motors Decipher Status.vi"("OS"=w1062) -> ("Status"=w1061:string)
                      n440 = property on="Theta (deg)" class="LVObjRef (strict)"() -> ("Value"=w1052:refnum<vi>)  [unwired: 2 in, 2 out]
                      n441 = property on="Status Theta" class="LVObjRef (strict)"() -> ("Value"=w1055:refnum<vi>)  [unwired: 2 in, 2 out]
                      n442 = property on="Property Node" class="Str"(reference=w1055, "Value"=w1061) -> ()  [unwired: 1 in, 2 out]
                      n443 = property on="Property Node" class="DigNum (strict)"(reference=w1052, "Value"=w1063) -> ()  [unwired: 1 in, 2 out]
                    }
                    n444 = call "Motors Stop.vi"("error in"=w1050, "Axis"=w1042, "VISA in"=w1051) -> ("error out"=w1048:errorcluster, "VISA out"=w1049:refnum<visa-resource-name>)
                  }
                }
              }
              frame #1 {
                n445 = property on="Property Node" class="Bool (strict)"(reference=w1072, "Value"=FALSE) -> ()  [unwired: 1 in, 2 out]
                n446 = property on="Property Node" class="Bool (strict)"(reference=w1073, "Value"=FALSE) -> ()  [unwired: 1 in, 2 out]
              }
            }
          }
        }
        n447 = property on="X Set Slew Speed?" class="LVObjRef (strict)"() -> ("Value"=w151:refnum<vi>)  [unwired: 2 in, 2 out]
        n448 = property on="Property Node" class="Bool (strict)"(reference=w151) -> (reference out=w174:refnum<vi>, "Value"=w178:bool)  [unwired: 1 in, 1 out]
        n449 = case shown="True" w178 {
          tunnel: [w976 w984] -> w274
          tunnel: w277 -> [w976 w985]
          tunnel: [w975 w988] -> w271
          tunnel: w270 -> [w975 w989]
          tunnel: w174 -> [_ w980]
          frame False {
          }
          frame True {
            n450 = property on="(mm/s)" class="LVObjRef (strict)"() -> ("Value"=w978:refnum<vi>)  [unwired: 2 in, 2 out]
            n451 = property on="Need to Update Motor Parameters" class="LVObjRef (strict)"() -> ("Value"=w977:refnum<vi>)  [unwired: 2 in, 2 out]
            n452 = property on="X Multiplier" class="LVObjRef (strict)"() -> ("Value"=w979:refnum<vi>)  [unwired: 2 in, 2 out]
            n453 = property on="Property Node" class="DigNum (strict)"(reference=w978) -> ("Value"=w982:dbl)  [unwired: 1 in, 2 out]
            n454 = property on="Property Node" class="DigNum (strict)"(reference=w979) -> ("Value"=w983:u32)  [unwired: 1 in, 2 out]
            n455 = property on="Property Node" class="Bool (strict)"(reference=w980, "Value"=FALSE) -> ()  [unwired: 1 in, 2 out]
            n456 = property on="Property Node" class="Bool (strict)"(reference=w977, "Value"=TRUE ("Need to Update Motor Parameters")) -> ()  [unwired: 1 in, 2 out]
            n457 = call "Motors Move Speed.vi"("Speed (mm or degree/sec)"=w982, "error in"=w989, "VISA in"=w985, "Axis"=u32 1, "Axis Multiplier"=w983) -> ("error out"=w988:errorcluster, "VISA out"=w984:refnum<visa-resource-name>)  [unwired: 5 in]
          }
        }
        n458 = property on="Y Set Slew Speed?" class="LVObjRef (strict)"() -> ("Value"=w150:refnum<vi>)  [unwired: 2 in, 2 out]
        n459 = property on="Property Node" class="Bool (strict)"(reference=w150) -> (reference out=w173:refnum<vi>, "Value"=w177:bool)  [unwired: 1 in, 1 out]
        n460 = case shown="True" w177 {
          tunnel: [w961 w970] -> w275
          tunnel: w274 -> [w961 w968]
          tunnel: [w960 w973] -> w272
          tunnel: w271 -> [w960 w974]
          tunnel: w173 -> [_ w965]
          frame False {
          }
          frame True {
            n461 = property on="Need to Update Motor Parameters" class="LVObjRef (strict)"() -> ("Value"=w962:refnum<vi>)  [unwired: 2 in, 2 out]
            n462 = property on="(mm/s) 2" class="LVObjRef (strict)"() -> ("Value"=w963:refnum<vi>)  [unwired: 2 in, 2 out]
            n463 = property on="Y Multiplier" class="LVObjRef (strict)"() -> ("Value"=w964:refnum<vi>)  [unwired: 2 in, 2 out]
            n464 = property on="Property Node" class="DigNum (strict)"(reference=w963) -> ("Value"=w967:dbl)  [unwired: 1 in, 2 out]
            n465 = property on="Property Node" class="DigNum (strict)"(reference=w964) -> ("Value"=w969:u32)  [unwired: 1 in, 2 out]
            n466 = property on="Property Node" class="Bool (strict)"(reference=w965, "Value"=FALSE) -> ()  [unwired: 1 in, 2 out]
            n467 = property on="Property Node" class="Bool (strict)"(reference=w962, "Value"=TRUE ("Need to Update Motor Parameters")) -> ()  [unwired: 1 in, 2 out]
            n468 = call "Motors Move Speed.vi"("Speed (mm or degree/sec)"=w967, "error in"=w974, "VISA in"=w968, "Axis"=u32 2, "Axis Multiplier"=w969) -> ("error out"=w973:errorcluster, "VISA out"=w970:refnum<visa-resource-name>)  [unwired: 5 in]
          }
        }
        n469 = property on="Z Set Slew Speed?" class="LVObjRef (strict)"() -> ("Value"=w149:refnum<vi>)  [unwired: 2 in, 2 out]
        n470 = property on="Property Node" class="Bool (strict)"(reference=w149) -> (reference out=w172:refnum<vi>, "Value"=w176:bool)  [unwired: 1 in, 1 out]
        n471 = case shown="True" w176 {
          tunnel: [w946 w955] -> w276
          tunnel: w275 -> [w946 w954]
          tunnel: [w945 w958] -> w273
          tunnel: w272 -> [w945 w959]
          tunnel: w172 -> [_ w950]
          frame False {
          }
          frame True {
            n472 = property on="Need to Update Motor Parameters" class="LVObjRef (strict)"() -> ("Value"=w947:refnum<vi>)  [unwired: 2 in, 2 out]
            n473 = property on="(mm/s) 3" class="LVObjRef (strict)"() -> ("Value"=w948:refnum<vi>)  [unwired: 2 in, 2 out]
            n474 = property on="Z Multiplier" class="LVObjRef (strict)"() -> ("Value"=w949:refnum<vi>)  [unwired: 2 in, 2 out]
            n475 = property on="Property Node" class="DigNum (strict)"(reference=w948) -> ("Value"=w952:dbl)  [unwired: 1 in, 2 out]
            n476 = property on="Property Node" class="DigNum (strict)"(reference=w949) -> ("Value"=w953:u32)  [unwired: 1 in, 2 out]
            n477 = property on="Property Node" class="Bool (strict)"(reference=w950, "Value"=FALSE) -> ()  [unwired: 1 in, 2 out]
            n478 = property on="Property Node" class="Bool (strict)"(reference=w947, "Value"=TRUE ("Need to Update Motor Parameters")) -> ()  [unwired: 1 in, 2 out]
            n479 = call "Motors Move Speed.vi"("Speed (mm or degree/sec)"=w952, "error in"=w959, "VISA in"=w954, "Axis"=u32 3, "Axis Multiplier"=w953) -> ("error out"=w958:errorcluster, "VISA out"=w955:refnum<visa-resource-name>)  [unwired: 5 in]
          }
        }
        n480 = property on="Theta Set Slew Speed?" class="LVObjRef (strict)"() -> ("Value"=w148:refnum<vi>)  [unwired: 2 in, 2 out]
        n481 = property on="Property Node" class="Bool (strict)"(reference=w148) -> (reference out=w171:refnum<vi>, "Value"=w175:bool)  [unwired: 1 in, 1 out]
        n482 = case shown="True" w175 {
          tunnel: [w931 w940] -> w268
          tunnel: w276 -> [w931 w939]
          tunnel: [w930 w941] -> w269
          tunnel: w273 -> [w930 w944]
          tunnel: w171 -> [_ w935]
          frame False {
          }
          frame True {
            n483 = property on="Theta Multiplier" class="LVObjRef (strict)"() -> ("Value"=w934:refnum<vi>)  [unwired: 2 in, 2 out]
            n484 = property on="Need to Update Motor Parameters" class="LVObjRef (strict)"() -> ("Value"=w932:refnum<vi>)  [unwired: 2 in, 2 out]
            n485 = property on="(degrees/s)" class="LVObjRef (strict)"() -> ("Value"=w933:refnum<vi>)  [unwired: 2 in, 2 out]
            n486 = property on="Property Node" class="DigNum (strict)"(reference=w933) -> ("Value"=w937:dbl)  [unwired: 1 in, 2 out]
            n487 = property on="Property Node" class="DigNum (strict)"(reference=w934) -> ("Value"=w938:u32)  [unwired: 1 in, 2 out]
            n488 = property on="Property Node" class="Bool (strict)"(reference=w935, "Value"=FALSE) -> ()  [unwired: 1 in, 2 out]
            n489 = property on="Property Node" class="Bool (strict)"(reference=w932, "Value"=TRUE ("Need to Update Motor Parameters")) -> ()  [unwired: 1 in, 2 out]
            n490 = call "Motors Move Speed.vi"("Speed (mm or degree/sec)"=w937, "error in"=w944, "VISA in"=w939, "Axis"=u32 4, "Axis Multiplier"=w938) -> ("error out"=w941:errorcluster, "VISA out"=w940:refnum<visa-resource-name>)  [unwired: 5 in]
          }
        }
        n491 = Quotient & Remainder(x=w246, y=4) -> (x-y*floor(x/y)=w266:i32)  [unwired: 1 out]
        n492 = case shown="3" w266 {
          tunnel: w269 -> [w770 w788 w805 w824]
          tunnel: w268 -> [w771 w789 w807 w825]
          tunnel: [w769 w786 w804 w823] -> w264
          tunnel: [w768 w787 w806 w822] -> w263
          frame 0, Default {
            n493 = property on="X Multiplier" class="LVObjRef (strict)"() -> ("Value"=w764:refnum<vi>)  [unwired: 2 in, 2 out]
            n494 = property on="Property Node" class="DigNum (strict)"(reference=w764) -> ("Value"=w767:u32)  [unwired: 1 in, 2 out]
            n495 = call "Motors Status.vi"("error in"=w770, "VISA in"=w771, "Axis"=1, "Axis Multiplier"=w767) -> ("error out"=w769:errorcluster, "VISA out"=w768:refnum<visa-resource-name>, "OS"=w777:i32, "Actual Position (mm or deg)"=w772:dbl)  [unwired: 3 in]
            n496 = call "Motors Decipher Status.vi"("OS"=w777) -> ("Status"=w776:string)
            n497 = Equal?(x=w776, y="Idle") -> (x = y?=w774:bool)
            n498 = case shown="False" w774 {
              tunnel: [TRUE FALSE] -> w773
              frame False {
              }
              frame True {
              }
            }
            n499 = property on="X Moving" class="LVObjRef (strict)"() -> ("Value"=w765:refnum<vi>)  [unwired: 2 in, 2 out]
            n500 = property on="X-Axis (mm)" class="LVObjRef (strict)"() -> ("Value"=w763:refnum<vi>)  [unwired: 2 in, 2 out]
            n501 = property on="Status X" class="LVObjRef (strict)"() -> ("Value"=w766:refnum<vi>)  [unwired: 2 in, 2 out]
            n502 = property on="Property Node" class="DigNum (strict)"(reference=w763, "Value"=w772) -> ()  [unwired: 1 in, 2 out]
            n503 = property on="Property Node" class="Bool (strict)"(reference=w765, "Value"=w773) -> ()  [unwired: 1 in, 2 out]
            n504 = property on="Property Node" class="Str"(reference=w766, "Value"=w776) -> ()  [unwired: 1 in, 2 out]
          }
          frame 1 {
            n505 = property on="Y Multiplier" class="LVObjRef (strict)"() -> ("Value"=w782:refnum<vi>)  [unwired: 2 in, 2 out]
            n506 = property on="Property Node" class="DigNum (strict)"(reference=w782) -> ("Value"=w785:u32)  [unwired: 1 in, 2 out]
            n507 = call "Motors Status.vi"("error in"=w788, "VISA in"=w789, "Axis"=2, "Axis Multiplier"=w785) -> ("error out"=w786:errorcluster, "VISA out"=w787:refnum<visa-resource-name>, "OS"=w794:i32, "Actual Position (mm or deg)"=w795:dbl)  [unwired: 3 in]
            n508 = call "Motors Decipher Status.vi"("OS"=w794) -> ("Status"=w792:string)
            n509 = Equal?(x=w792, y="Idle") -> (x = y?=w791:bool)
            n510 = case shown="False" w791 {
              tunnel: [TRUE FALSE] -> w790
              frame False {
              }
              frame True {
              }
            }
            n511 = property on="Y Moving" class="LVObjRef (strict)"() -> ("Value"=w784:refnum<vi>)  [unwired: 2 in, 2 out]
            n512 = property on="Y-Axis (mm)" class="LVObjRef (strict)"() -> ("Value"=w781:refnum<vi>)  [unwired: 2 in, 2 out]
            n513 = property on="Status Y" class="LVObjRef (strict)"() -> ("Value"=w783:refnum<vi>)  [unwired: 2 in, 2 out]
            n514 = property on="Property Node" class="DigNum (strict)"(reference=w781, "Value"=w795) -> ()  [unwired: 1 in, 2 out]
            n515 = property on="Property Node" class="Bool (strict)"(reference=w784, "Value"=w790) -> ()  [unwired: 1 in, 2 out]
            n516 = property on="Property Node" class="Str"(reference=w783, "Value"=w792) -> ()  [unwired: 1 in, 2 out]
          }
          frame 2 {
            n517 = property on="Z Multiplier" class="LVObjRef (strict)"() -> ("Value"=w801:refnum<vi>)  [unwired: 2 in, 2 out]
            n518 = property on="Property Node" class="DigNum (strict)"(reference=w801) -> ("Value"=w803:u32)  [unwired: 1 in, 2 out]
            n519 = call "Motors Status.vi"("error in"=w805, "VISA in"=w807, "Axis"=3, "Axis Multiplier"=w803) -> ("error out"=w804:errorcluster, "VISA out"=w806:refnum<visa-resource-name>, "OS"=w812:i32, "Actual Position (mm or deg)"=w813:dbl)  [unwired: 3 in]
            n520 = call "Motors Decipher Status.vi"("OS"=w812) -> ("Status"=w810:string)
            n521 = Equal?(x=w810, y="Idle") -> (x = y?=w809:bool)
            n522 = case shown="False" w809 {
              tunnel: [TRUE FALSE] -> w808
              frame False {
              }
              frame True {
              }
            }
            n523 = property on="Z Moving" class="LVObjRef (strict)"() -> ("Value"=w800:refnum<vi>)  [unwired: 2 in, 2 out]
            n524 = property on="Z-Axis (mm)" class="LVObjRef (strict)"() -> ("Value"=w799:refnum<vi>)  [unwired: 2 in, 2 out]
            n525 = property on="Status Z" class="LVObjRef (strict)"() -> ("Value"=w802:refnum<vi>)  [unwired: 2 in, 2 out]
            n526 = property on="Property Node" class="DigNum (strict)"(reference=w799, "Value"=w813) -> ()  [unwired: 1 in, 2 out]
            n527 = property on="Property Node" class="Str"(reference=w802, "Value"=w810) -> ()  [unwired: 1 in, 2 out]
            n528 = property on="Property Node" class="Bool (strict)"(reference=w800, "Value"=w808) -> ()  [unwired: 1 in, 2 out]
          }
          frame 3 {
            n529 = property on="Theta Multiplier" class="LVObjRef (strict)"() -> ("Value"=w819:refnum<vi>)  [unwired: 2 in, 2 out]
            n530 = property on="Property Node" class="DigNum (strict)"(reference=w819) -> ("Value"=w821:u32)  [unwired: 1 in, 2 out]
            n531 = call "Motors Status.vi"("error in"=w824, "VISA in"=w825, "Axis"=4, "Axis Multiplier"=w821) -> ("error out"=w823:errorcluster, "VISA out"=w822:refnum<visa-resource-name>, "OS"=w830:i32, "Actual Position (mm or deg)"=w831:dbl)  [unwired: 3 in]
            n532 = call "Motors Decipher Status.vi"("OS"=w830) -> ("Status"=w828:string)
            n533 = Equal?(x=w828, y="Idle") -> (x = y?=w827:bool)
            n534 = case shown="True" w827 {
              tunnel: [TRUE FALSE] -> w826
              frame False {
              }
              frame True {
              }
            }
            n535 = property on="Theta (deg)" class="LVObjRef (strict)"() -> ("Value"=w817:refnum<vi>)  [unwired: 2 in, 2 out]
            n536 = property on="Status Theta" class="LVObjRef (strict)"() -> ("Value"=w820:refnum<vi>)  [unwired: 2 in, 2 out]
            n537 = property on="Theta Moving" class="LVObjRef (strict)"() -> ("Value"=w818:refnum<vi>)  [unwired: 2 in, 2 out]
            n538 = property on="Property Node" class="DigNum (strict)"(reference=w817, "Value"=w831) -> ()  [unwired: 1 in, 2 out]
            n539 = property on="Property Node" class="Str"(reference=w820, "Value"=w828) -> ()  [unwired: 1 in, 2 out]
            n540 = property on="Property Node" class="Bool (strict)"(reference=w818, "Value"=w826) -> ()  [unwired: 1 in, 2 out]
          }
        }
        n541 = property on="Go To Saved Position?" class="LVObjRef (strict)"() -> ("Value"=w126:refnum<vi>)  [unwired: 2 in, 2 out]
        n542 = property on="Property Node" class="Bool (strict)"(reference=w126) -> (reference out=w169:refnum<vi>, "Value"=w170:bool)  [unwired: 1 in, 1 out]
        n543 = case shown="True" w170 {
          tunnel: w264 -> [w724 w735]
          tunnel: w263 -> [w723 w741]
          tunnel: [w724 w754] -> w262
          tunnel: [w723 w753] -> w261
          tunnel: w169 -> [_ w732]
          frame False {
          }
          frame True {
            w751 = 4 ("index (row)")
            w749 = 3 ("index (row)")
            w746 = 2 ("index (row)")
            w743 = 1 ("index (row)")
            n544 = property on="Property Node" class="Bool (strict)"(reference=w732, "Value"=FALSE) -> ()  [unwired: 1 in, 2 out]
            n545 = property on="Theta Multiplier" class="LVObjRef (strict)"() -> ("Value"=w727:refnum<vi>)  [unwired: 2 in, 2 out]
            n546 = property on="Defined Positions" class="LVObjRef (strict)"() -> ("Value"=w725:refnum<vi>)  [unwired: 2 in, 2 out]
            n547 = property on="Saved Positions" class="LVObjRef (strict)"() -> ("Value"=w726:refnum<vi>)  [unwired: 2 in, 2 out]
            n548 = property on="Z Multiplier" class="LVObjRef (strict)"() -> ("Value"=w728:refnum<vi>)  [unwired: 2 in, 2 out]
            n549 = property on="Y Multiplier" class="LVObjRef (strict)"() -> ("Value"=w729:refnum<vi>)  [unwired: 2 in, 2 out]
            n550 = property on="X Multiplier" class="LVObjRef (strict)"() -> ("Value"=w730:refnum<vi>)  [unwired: 2 in, 2 out]
            n551 = property on="Property Node" class="DigNum (strict)"(reference=w727) -> ("Value"=w737:u32)  [unwired: 1 in, 2 out]
            n552 = property on="Property Node" class="DigNum (strict)"(reference=w728) -> ("Value"=w738:u32)  [unwired: 1 in, 2 out]
            n553 = property on="Property Node" class="DigNum (strict)"(reference=w729) -> ("Value"=w739:u32)  [unwired: 1 in, 2 out]
            n554 = property on="Property Node" class="DigNum (strict)"(reference=w730) -> ("Value"=w740:u32)  [unwired: 1 in, 2 out]
            n555 = property on="Property Node" class="Path"(reference=w726) -> ("Value"=w736:path)  [unwired: 1 in, 2 out]
            n556 = property on="Property Node" class="LstBox (strict)"(reference=w725) -> ("Value"=w731:i32)  [unwired: 1 in, 2 out]
            n557 = call "Motors Position Load.vi"("error in"=w735, "file path"=w736) -> ("error out"=w734:errorcluster, "Positions"=w757:string[][])
            n558 = Index Array(array=w757, index (row)=w751, index (col)=w731) -> (element=w758:string)
            n559 = Index Array(array=w757, index (row)=w749, index (col)=w731) -> (element=w759:string)
            n560 = Index Array(array=w757, index (row)=w746, index (col)=w731) -> (element=w761:string)
            n561 = Index Array(array=w757, index (row)=w743, index (col)=w731) -> (element=w762:string)
            n562 = Fract/Exp String To Number(string=w758) -> (number=w752:dbl)  [unwired: 3 in, 1 out]
            n563 = Fract/Exp String To Number(string=w759) -> (number=w748:dbl)  [unwired: 3 in, 1 out]
            n564 = Fract/Exp String To Number(string=w761) -> (number=w745:dbl)  [unwired: 3 in, 1 out]
            n565 = Fract/Exp String To Number(string=w762) -> (number=w742:dbl)  [unwired: 3 in, 1 out]
            n566 = call "Motors Move Absolute.vi"("Axis Multiplier"=w740, "Axis"=w743, "error in"=w734, "VISA in"=w741, "Position (mm or degree)"=w742) -> ("error out"=w760:errorcluster, "VISA out"=w744:refnum<visa-resource-name>)  [unwired: 5 in]
            n567 = call "Motors Move Absolute.vi"("Axis Multiplier"=w739, "Axis"=w746, "error in"=w760, "VISA in"=w744, "Position (mm or degree)"=w745) -> ("error out"=w756:errorcluster, "VISA out"=w747:refnum<visa-resource-name>)  [unwired: 5 in]
            n568 = call "Motors Move Absolute.vi"("Axis Multiplier"=w738, "Axis"=w749, "error in"=w756, "VISA in"=w747, "Position (mm or degree)"=w748) -> ("error out"=w755:errorcluster, "VISA out"=w750:refnum<visa-resource-name>)  [unwired: 5 in]
            n569 = call "Motors Move Absolute.vi"("Axis Multiplier"=w737, "Axis"=w751, "error in"=w755, "VISA in"=w750, "Position (mm or degree)"=w752) -> ("error out"=w754:errorcluster, "VISA out"=w753:refnum<visa-resource-name>)  [unwired: 5 in]
          }
        }
        n570 = property on="Need to Update Motor Parameters" class="LVObjRef (strict)"() -> ("Value"=w145:refnum<vi>)  [unwired: 2 in, 2 out]
        n571 = property on="Property Node" class="Bool (strict)"(reference=w145) -> (reference out=w167:refnum<vi>, "Value"=w267:bool)  [unwired: 1 in, 1 out]
        n572 = case shown="True" w267 {
          tunnel: w262 -> [w836 w843]
          tunnel: w261 -> [w835 w844]
          tunnel: [w835 w842] -> w122
          tunnel: [w836 w841] -> w125
          tunnel: w168 -> [_ w840]
          tunnel: w167 -> [_ w839]
          frame False {
          }
          frame True {
            n573 = flat-sequence {
              tunnel: w840 -> [w847]
              tunnel: [w846] -> w838
              tunnel: w844 -> [w882]
              tunnel: w843 -> [w881]
              tunnel: [w880] -> w842
              tunnel: [w879] -> w841
              tunnel: w838 -> [w873]
              tunnel: [w873] -> w837
              tunnel: w837 -> [w928]
              frame #0 {
                n574 = call <vilib>:"Set Busy.vi"() -> ()  [unwired: 10 in, 2 out]
                n575 = property on="Property Node" class="Str"(reference=w847, "Value"="Updating Motor Parameters\nThis Should Take About 5 Seconds" ("Status Theta")) -> (reference out=w846:refnum<vi>)  [unwired: 1 in, 1 out]
              }
              frame #1 {
                n576 = call "Motors Status Verbose.vi"("Axis"=1, "VISA in"=w882, "error in"=w881) -> ("Slew Speed (mm or deg/s)"=w898:dbl, "Jogger Normal Speed (mm or deg/s)"=w899:dbl, "Jogger Fast Speed (mm or deg/s)"=w900:dbl, "Actual Position (mm or deg)"=w915:dbl, "OS"=w889:i32, "Mode"=→"X Action":string, "VISA out"=w904:refnum<visa-resource-name>, "Creep Speed (mm or deg/s)"=w877:dbl, "error out"=w886:errorcluster)  [unwired: 4 in]
                n577 = property on="X Slew Speed (mm or degree/s)" class="LVObjRef (strict)"() -> ("Value"=w860:refnum<vi>)  [unwired: 2 in, 2 out]
                n578 = property on="Property Node" class="DigNum (strict)"(reference=w860, "Value"=w898) -> ()  [unwired: 1 in, 2 out]
                n579 = property on="Property Node" class="DigNum (strict)"(reference=w860, "Minimum"=w877) -> ()  [unwired: 1 in, 2 out]
                n580 = property on="X Jogger Fast Speed" class="LVObjRef (strict)"() -> ("Value"=w861:refnum<vi>)  [unwired: 2 in, 2 out]
                n581 = property on="X-Axis (mm)" class="LVObjRef (strict)"() -> ("Value"=w856:refnum<vi>)  [unwired: 2 in, 2 out]
                n582 = property on="X Jogger Normal Speed" class="LVObjRef (strict)"() -> ("Value"=w862:refnum<vi>)  [unwired: 2 in, 2 out]
                n583 = property on="Property Node" class="DigNum (strict)"(reference=w862, "Value"=w899) -> ()  [unwired: 1 in, 2 out]
                n584 = property on="Property Node" class="DigNum (strict)"(reference=w861, "Value"=w900) -> ()  [unwired: 1 in, 2 out]
                n585 = property on="Property Node" class="DigNum (strict)"(reference=w856, "Value"=w915) -> ()  [unwired: 1 in, 2 out]
                n586 = call "Motors Status Verbose.vi"("Axis"=2, "VISA in"=w904, "error in"=w886) -> ("Slew Speed (mm or deg/s)"=w901:dbl, "Jogger Normal Speed (mm or deg/s)"=w902:dbl, "Jogger Fast Speed (mm or deg/s)"=w903:dbl, "Actual Position (mm or deg)"=w916:dbl, "OS"=w890:i32, "Mode"=→"Y Action":string, "VISA out"=w905:refnum<visa-resource-name>, "Creep Speed (mm or deg/s)"=w876:dbl, "error out"=w887:errorcluster)  [unwired: 4 in]
                n587 = call "Motors Decipher Status.vi"("OS"=w889) -> ("Status"=w925:string)
                n588 = property on="Y Slew Speed (mm or degree/s)" class="LVObjRef (strict)"() -> ("Value"=w857:refnum<vi>)  [unwired: 2 in, 2 out]
                n589 = property on="Property Node" class="DigNum (strict)"(reference=w857, "Value"=w901) -> ()  [unwired: 1 in, 2 out]
                n590 = property on="Property Node" class="DigNum (strict)"(reference=w857, "Minimum"=w876) -> ()  [unwired: 1 in, 2 out]
                n591 = Not Equal?(x=w925, y="Idle") -> (x != y?=w907:bool)
                n592 = property on="Status X" class="LVObjRef (strict)"() -> ("Value"=w864:refnum<vi>)  [unwired: 2 in, 2 out]
                n593 = property on="Y Jogger Fast Speed" class="LVObjRef (strict)"() -> ("Value"=w870:refnum<vi>)  [unwired: 2 in, 2 out]
                n594 = property on="Y-Axis (mm)" class="LVObjRef (strict)"() -> ("Value"=w858:refnum<vi>)  [unwired: 2 in, 2 out]
                n595 = property on="Y Jogger Normal Speed" class="LVObjRef (strict)"() -> ("Value"=w866:refnum<vi>)  [unwired: 2 in, 2 out]
                n596 = property on="Property Node" class="Str"(reference=w864, "Value"=w925) -> ()  [unwired: 1 in, 2 out]
                n597 = property on="Property Node" class="DigNum (strict)"(reference=w866, "Value"=w902) -> ()  [unwired: 1 in, 2 out]
                n598 = property on="Property Node" class="DigNum (strict)"(reference=w870, "Value"=w903) -> ()  [unwired: 1 in, 2 out]
                n599 = property on="Property Node" class="DigNum (strict)"(reference=w858, "Value"=w916) -> ()  [unwired: 1 in, 2 out]
                n600 = call "Motors Status Verbose.vi"("Axis"=3, "VISA in"=w905, "error in"=w887) -> ("Slew Speed (mm or deg/s)"=w914:dbl, "Jogger Normal Speed (mm or deg/s)"=w913:dbl, "Jogger Fast Speed (mm or deg/s)"=w912:dbl, "Actual Position (mm or deg)"=w911:dbl, "OS"=w891:i32, "Mode"=→"Z Action":string, "VISA out"=w906:refnum<visa-resource-name>, "Creep Speed (mm or deg/s)"=w875:dbl, "error out"=w888:errorcluster)  [unwired: 4 in]
                n601 = call "Motors Decipher Status.vi"("OS"=w890) -> ("Status"=w917:string)
                n602 = property on="X Moving" class="LVObjRef (strict)"() -> ("Value"=w863:refnum<vi>)  [unwired: 2 in, 2 out]
                n603 = property on="Z Slew Speed (mm or degree/s)" class="LVObjRef (strict)"() -> ("Value"=w859:refnum<vi>)  [unwired: 2 in, 2 out]
                n604 = property on="Property Node" class="Bool (strict)"(reference=w863, "Value"=w907) -> ()  [unwired: 1 in, 2 out]
                n605 = property on="Property Node" class="DigNum (strict)"(reference=w859, "Value"=w914) -> ()  [unwired: 1 in, 2 out]
                n606 = property on="Property Node" class="DigNum (strict)"(reference=w859, "Minimum"=w875) -> ()  [unwired: 1 in, 2 out]
                n607 = Not Equal?(x=w917, y="Idle") -> (x != y?=w908:bool)
                n608 = property on="Status Y" class="LVObjRef (strict)"() -> ("Value"=w853:refnum<vi>)  [unwired: 2 in, 2 out]
                n609 = property on="Z Jogger Fast Speed" class="LVObjRef (strict)"() -> ("Value"=w868:refnum<vi>)  [unwired: 2 in, 2 out]
                n610 = property on="Z-Axis (mm)" class="LVObjRef (strict)"() -> ("Value"=w872:refnum<vi>)  [unwired: 2 in, 2 out]
                n611 = property on="Z Jogger Normal Speed" class="LVObjRef (strict)"() -> ("Value"=w869:refnum<vi>)  [unwired: 2 in, 2 out]
                n612 = property on="Property Node" class="Str"(reference=w853, "Value"=w917) -> ()  [unwired: 1 in, 2 out]
                n613 = property on="Property Node" class="DigNum (strict)"(reference=w869, "Value"=w913) -> ()  [unwired: 1 in, 2 out]
                n614 = property on="Property Node" class="DigNum (strict)"(reference=w868, "Value"=w912) -> ()  [unwired: 1 in, 2 out]
                n615 = property on="Property Node" class="DigNum (strict)"(reference=w872, "Value"=w911) -> ()  [unwired: 1 in, 2 out]
                n616 = call "Motors Status Verbose.vi"("Axis"=4, "VISA in"=w906, "error in"=w888) -> ("Slew Speed (mm or deg/s)"=w920:dbl, "Jogger Normal Speed (mm or deg/s)"=w921:dbl, "Jogger Fast Speed (mm or deg/s)"=w922:dbl, "Actual Position (mm or deg)"=w923:dbl, "OS"=w892:i32, "Mode"=→"Theta Action":string, "VISA out"=w880:refnum<visa-resource-name>, "Creep Speed (mm or deg/s)"=w874:dbl, "error out"=w879:errorcluster)  [unwired: 4 in]
                n617 = call "Motors Decipher Status.vi"("OS"=w891) -> ("Status"=w919:string)
                n618 = property on="Y Moving" class="LVObjRef (strict)"() -> ("Value"=w871:refnum<vi>)  [unwired: 2 in, 2 out]
                n619 = property on="Theta Slew Speed (mm or degree/s)" class="LVObjRef (strict)"() -> ("Value"=w850:refnum<vi>)  [unwired: 2 in, 2 out]
                n620 = property on="Property Node" class="Bool (strict)"(reference=w871, "Value"=w908) -> ()  [unwired: 1 in, 2 out]
                n621 = property on="Property Node" class="DigNum (strict)"(reference=w850, "Value"=w920) -> ()  [unwired: 1 in, 2 out]
                n622 = property on="Property Node" class="DigNum (strict)"(reference=w850, "Minimum"=w874) -> ()  [unwired: 1 in, 2 out]
                n623 = Not Equal?(x=w919, y="Idle") -> (x != y?=w909:bool)
                n624 = property on="Theta Jogger Fast Speed" class="LVObjRef (strict)"() -> ("Value"=w852:refnum<vi>)  [unwired: 2 in, 2 out]
                n625 = property on="Theta (deg)" class="LVObjRef (strict)"() -> ("Value"=w855:refnum<vi>)  [unwired: 2 in, 2 out]
                n626 = property on="Status Z" class="LVObjRef (strict)"() -> ("Value"=w854:refnum<vi>)  [unwired: 2 in, 2 out]
                n627 = property on="Theta Jogger Normal Speed" class="LVObjRef (strict)"() -> ("Value"=w851:refnum<vi>)  [unwired: 2 in, 2 out]
                n628 = property on="Property Node" class="Str"(reference=w854, "Value"=w919) -> ()  [unwired: 1 in, 2 out]
                n629 = property on="Property Node" class="DigNum (strict)"(reference=w851, "Value"=w921) -> ()  [unwired: 1 in, 2 out]
                n630 = property on="Property Node" class="DigNum (strict)"(reference=w852, "Value"=w922) -> ()  [unwired: 1 in, 2 out]
                n631 = property on="Property Node" class="DigNum (strict)"(reference=w855, "Value"=w923) -> ()  [unwired: 1 in, 2 out]
                n632 = call "Motors Decipher Status.vi"("OS"=w892) -> ("Status"=w927:string)
                n633 = property on="Z Moving" class="LVObjRef (strict)"() -> ("Value"=w865:refnum<vi>)  [unwired: 2 in, 2 out]
                n634 = property on="Property Node" class="Bool (strict)"(reference=w865, "Value"=w909) -> ()  [unwired: 1 in, 2 out]
                n635 = Not Equal?(x=w927, y="Idle") -> (x != y?=w910:bool)
                n636 = property on="Status Theta" class="LVObjRef (strict)"() -> ("Value"=w867:refnum<vi>)  [unwired: 2 in, 2 out]
                n637 = property on="Property Node" class="Str"(reference=w867, "Value"=w927) -> ()  [unwired: 1 in, 2 out]
                n638 = property on="Theta Moving" class="LVObjRef (strict)"() -> ("Value"=w849:refnum<vi>)  [unwired: 2 in, 2 out]
                n639 = property on="Property Node" class="Bool (strict)"(reference=w849, "Value"=w910) -> ()  [unwired: 1 in, 2 out]
              }
              frame #2 {
                n640 = call <vilib>:"Unset Busy.vi"() -> ()  [unwired: 11 in, 1 out]
                n641 = property on="Property Node" class="Str"(reference=w928, "Value"="Running" ("Status Theta")) -> ()  [unwired: 1 in, 2 out]
              }
            }
            n642 = property on="Property Node" class="Bool (strict)"(reference=w839, "Value"=FALSE ("Need to Update Motor Parameters")) -> ()  [unwired: 1 in, 2 out]
          }
        }
        n643 = property on="Property Node" class="Clust (strict)"(reference=w124, "Value"=w125) -> ()  [unwired: 1 in, 2 out]
        "Loop i" <- w246
      }
    }
  }
  n644 = property on="Property Node" class="Clust (strict)"(reference=w16) -> (reference out=w15:refnum<vi>, "Value"=w18:errorcluster)  [unwired: 1 in, 1 out]
  n645 = call "Motors Close.vi"("error in"=w18, "VISA in"=w1) -> ("error out"=w17:errorcluster)  [unwired: 1 in]
  n646 = property on="Property Node" class="Clust (strict)"(reference=w15, "Value"=w17) -> ()  [unwired: 1 in, 2 out]
